vi "Motors Modular Bk.vi"(0 "Enable Motors":refnum<vi>, 1 "Cluster":T1, 2 "Motors Visa Ref":refnum<visa-resource-name>="COM7") -> ()   [LabVIEW 2010]
panel:
  in  "Enable Motors":bool
  out "Theta Action":string
  out "Z Action":string
  out "Y Action":string
  out "X Action":string
  in  "Steps to deactivate hard limit after finding datums":dbl=1000.0
  out "Loop i":i32
types:
  T1 = cluster{"Stop X?":refnum<vi>, "Stop Y?":refnum<vi>, "Stop Z?":refnum<vi>, "Stop Theta?":refnum<vi>, "Backlash?":refnum<vi>, "Backlash X":refnum<vi>, "Backlash Y":refnum<vi>, "Backlash Z":refnum<vi>, "Backlash Theta":refnum<vi>, "Manual IO?":refnum<vi>, "Manual Communication is Active\n(Close Before Ending Program)":refnum<vi>, "Reset Motors?":refnum<vi>, "Set Jogger?":refnum<vi>, "Normal":refnum<vi>, "Fast":refnum<vi>, "Jogger Axis":refnum<vi>, "Redefine Origin as Current Location?":refnum<vi>, "Save Current Motor Parameters?":refnum<vi>, "Find Datums Nearest Hard Limits?":refnum<vi>, "Saved Limits":refnum<vi>, "Use Datums Nearest Hard Limits to Reset Origin?":refnum<vi>, "X Go?":refnum<vi>, "Y Go?":refnum<vi>, "Z Go?":refnum<vi>, "Theta Go?":refnum<vi>, "Jog-Mode":refnum<vi>, "x+?":refnum<vi>, "x-?":refnum<vi>, "y+?":refnum<vi>, "y-?":refnum<vi>, "z+?":refnum<vi>, "z-?":refnum<vi>, "theta+?":refnum<vi>, "theta-?":refnum<vi>, "X Set Slew Speed?":refnum<vi>, "(mm/s)":refnum<vi>, "Y Set Slew Speed?":refnum<vi>, "(mm/s)":refnum<vi>, "Z Set Slew Speed?":refnum<vi>, "(mm/s)":refnum<vi>, "Theta Set Slew Speed?":refnum<vi>, "(degrees/s)":refnum<vi>, "Go To Saved Position?":refnum<vi>, "Defined Positions":refnum<vi>, "Need to Update Motor Parameters":refnum<vi>, "X Jogger Normal Speed":refnum<vi>, "X Jogger Fast Speed":refnum<vi>, "Y Jogger Normal Speed":refnum<vi>, "Y Jogger Fast Speed":refnum<vi>, "Z Jogger Normal Speed":refnum<vi>, "Z Jogger Fast Speed":refnum<vi>, "Theta Jogger Normal Speed":refnum<vi>, "Theta Jogger Fast Speed":refnum<vi>, "X Moving":refnum<vi>, "Y Moving":refnum<vi>, "Z Moving":refnum<vi>, "Theta Moving":refnum<vi>, "X Slew Speed (mm or degree/s)":refnum<vi>, "Y Slew Speed (mm or degree/s)":refnum<vi>, "Z Slew Speed (mm or degree/s)":refnum<vi>, "Theta Slew Speed (mm or degree/s)":refnum<vi>, "X-Axis (mm)":refnum<vi>, "Y-Axis (mm)":refnum<vi>, "Z-Axis (mm)":refnum<vi>, "Theta (deg)":refnum<vi>, "X Multiplier":refnum<vi>, "Y Multiplier":refnum<vi>, "Z Multiplier":refnum<vi>, "Theta Multiplier":refnum<vi>, "Motors Online":refnum<vi>, "Motors Status":refnum<vi>, "Status X":refnum<vi>, "Status Y":refnum<vi>, "Status Z":refnum<vi>, "Status Theta":refnum<vi>, "Motors error":refnum<vi>, "QUIT":refnum<vi>, "EMERGENCY":refnum<vi>, "X Go To":refnum<vi>, "Y Go To":refnum<vi>, "Z Go To":refnum<vi>, "Theta Go To":refnum<vi>, "Delta X (mm)":refnum<vi>, "Delta Y (mm)":refnum<vi>, "Delta Z (mm)":refnum<vi>, "Delta Theta (deg)":refnum<vi>, "X Speed (mm/s)":refnum<vi>, "Y Speed (mm/s)":refnum<vi>, "Z Speed (mm/s)":refnum<vi>, "Theta Speed (deg/s)":refnum<vi>, "x+":refnum<vi>, "x-":refnum<vi>, "y+":refnum<vi>, "y-":refnum<vi>, "z+":refnum<vi>, "z-":refnum<vi>, "theta+":refnum<vi>, "theta-":refnum<vi>, "Saved Positions":refnum<vi>}
  T2 = cluster{"Stop X?":refnum<vi>, "Stop Y?":refnum<vi>, "Stop Z?":refnum<vi>, "Stop Theta?":refnum<vi>}
  T3 = cluster{"Backlash?":refnum<vi>, "Backlash X":refnum<vi>, "Backlash Y":refnum<vi>, "Backlash Z":refnum<vi>, "Backlash Theta":refnum<vi>}
  T4 = cluster{"EMERGENCY":refnum<vi>, "Manual IO?":refnum<vi>, "Manual Communication is Active\n(Close Before Ending Program)":refnum<vi>, "Reset Motors?":refnum<vi>}
  T5 = cluster{"Redefine Origin as Current Location?":refnum<vi>, "Save Current Motor Parameters?":refnum<vi>}
  T6 = cluster{"X Set Slew Speed?":refnum<vi>, "(mm/s)":refnum<vi>, "Y Set Slew Speed?":refnum<vi>, "(mm/s)":refnum<vi>, "Z Set Slew Speed?":refnum<vi>, "(mm/s)":refnum<vi>, "Theta Set Slew Speed?":refnum<vi>, "(degrees/s)":refnum<vi>, "Need to Update Motor Parameters":refnum<vi>, "X Multiplier":refnum<vi>, "Y Multiplier":refnum<vi>, "Z Multiplier":refnum<vi>, "Theta Multiplier":refnum<vi>}
  T7 = cluster{"Set Jogger?":refnum<vi>, "Normal":refnum<vi>, "Fast":refnum<vi>, "Jogger Axis":refnum<vi>, "X Multiplier":refnum<vi>, "Y Multiplier":refnum<vi>, "Z Multiplier":refnum<vi>, "Theta Multiplier":refnum<vi>, "Need to Update Motor Parameters":refnum<vi>}
  T8 = cluster{"Need to Update Motor Parameters":refnum<vi>, "X Jogger Normal Speed":refnum<vi>, "X Jogger Fast Speed":refnum<vi>, "X Slew Speed (mm or degree/s)":refnum<vi>, "X-Axis (mm)":refnum<vi>, "Status X":refnum<vi>, "X Moving":refnum<vi>}
  T9 = cluster{"Y Slew Speed (mm or degree/s)":refnum<vi>, "Y Jogger Normal Speed":refnum<vi>, "Y Jogger Fast Speed":refnum<vi>, "Y-Axis (mm)":refnum<vi>, "Status Y":refnum<vi>, "Y Moving":refnum<vi>}
  T10 = cluster{"Z Slew Speed (mm or degree/s)":refnum<vi>, "Z Jogger Normal Speed":refnum<vi>, "Z Jogger Fast Speed":refnum<vi>, "Z-Axis (mm)":refnum<vi>, "Status Z":refnum<vi>, "Z Moving":refnum<vi>}
  T11 = cluster{"Theta Slew Speed (mm or degree/s)":refnum<vi>, "Theta Jogger Normal Speed":refnum<vi>, "Theta Jogger Fast Speed":refnum<vi>, "Theta (deg)":refnum<vi>, "Status Theta":refnum<vi>, "Theta Moving":refnum<vi>}
  T12 = cluster{"Find Datums Nearest Hard Limits?":refnum<vi>, "X Multiplier":refnum<vi>, "Y Multiplier":refnum<vi>, "Z Multiplier":refnum<vi>, "Theta Multiplier":refnum<vi>, "X-Axis (mm)":refnum<vi>, "Y-Axis (mm)":refnum<vi>, "Z-Axis (mm)":refnum<vi>, "Theta (deg)":refnum<vi>, "Status X":refnum<vi>, "Status Y":refnum<vi>, "Status Z":refnum<vi>, "Status Theta":refnum<vi>, "X Moving":refnum<vi>, "Y Moving":refnum<vi>, "Z Moving":refnum<vi>, "Theta Moving":refnum<vi>, "Saved Limits":refnum<vi>}
  T13 = cluster{"Status X":refnum<vi>, "X-Axis (mm)":refnum<vi>, "X Multiplier":refnum<vi>, "X Moving":refnum<vi>, "Status Y":refnum<vi>, "Y-Axis (mm)":refnum<vi>, "Y Multiplier":refnum<vi>, "Y Moving":refnum<vi>, "Status Z":refnum<vi>, "Z-Axis (mm)":refnum<vi>, "Z Multiplier":refnum<vi>, "Z Moving":refnum<vi>, "Status Theta":refnum<vi>, "Theta (deg)":refnum<vi>, "Theta Multiplier":refnum<vi>, "Theta Moving":refnum<vi>}
  T14 = cluster{"Use Datums Nearest Hard Limits to Reset Origin?":refnum<vi>, "X Multiplier":refnum<vi>, "Y Multiplier":refnum<vi>, "Z Multiplier":refnum<vi>, "Theta Multiplier":refnum<vi>, "X-Axis (mm)":refnum<vi>, "Y-Axis (mm)":refnum<vi>, "Z-Axis (mm)":refnum<vi>, "Theta (deg)":refnum<vi>, "Status X":refnum<vi>, "Status Y":refnum<vi>, "Status Z":refnum<vi>, "Status Theta":refnum<vi>}
  T15 = cluster{"X Go?":refnum<vi>, "X Multiplier":refnum<vi>, "X Go To":refnum<vi>, "Y Go?":refnum<vi>, "Y Multiplier":refnum<vi>, "Y Go To":refnum<vi>, "Z Go?":refnum<vi>, "Z Multiplier":refnum<vi>, "Z Go To":refnum<vi>, "Theta Go?":refnum<vi>, "Theta Multiplier":refnum<vi>, "Theta Go To":refnum<vi>}
  T16 = cluster{"Jog-Mode":refnum<vi>, "x+?":refnum<vi>, "x-?":refnum<vi>, "X Moving":refnum<vi>, "X Multiplier":refnum<vi>, "Delta X (mm)":refnum<vi>, "X Speed (mm/s)":refnum<vi>, "x+":refnum<vi>, "x-":refnum<vi>, "X-Axis (mm)":refnum<vi>, "Status X":refnum<vi>}
  T17 = cluster{"Jog-Mode":refnum<vi>, "y+?":refnum<vi>, "y-?":refnum<vi>, "Y Moving":refnum<vi>, "Delta Y (mm)":refnum<vi>, "Y Multiplier":refnum<vi>, "y+":refnum<vi>, "y-":refnum<vi>, "Y-Axis (mm)":refnum<vi>, "Status Y":refnum<vi>, "Y Speed (mm/s)":refnum<vi>}
  T18 = cluster{"Go To Saved Position?":refnum<vi>, "Defined Positions":refnum<vi>, "X Multiplier":refnum<vi>, "Y Multiplier":refnum<vi>, "Z Multiplier":refnum<vi>, "Theta Multiplier":refnum<vi>, "Saved Positions":refnum<vi>}
  T19 = cluster{"Jog-Mode":refnum<vi>, "z+?":refnum<vi>, "z-?":refnum<vi>, "Z Speed (mm/s)":refnum<vi>, "Delta Z (mm)":refnum<vi>, "Z Multiplier":refnum<vi>, "Z-Axis (mm)":refnum<vi>, "Status Z":refnum<vi>, "z+":refnum<vi>, "z-":refnum<vi>, "Z Moving":refnum<vi>}
  T20 = cluster{"Jog-Mode":refnum<vi>, "theta+?":refnum<vi>, "theta-?":refnum<vi>, "Theta Speed (deg/s)":refnum<vi>, "Delta Theta (deg)":refnum<vi>, "Theta Multiplier":refnum<vi>, "Theta (deg)":refnum<vi>, "Status Theta":refnum<vi>, "theta+":refnum<vi>, "theta-":refnum<vi>, "Theta Moving":refnum<vi>}
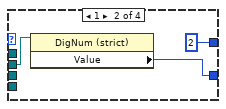
[diagram p3: hidden frame]
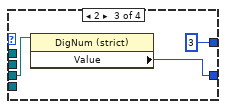
[diagram p4: hidden frame]
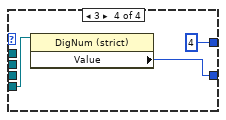
[diagram p5: hidden frame]
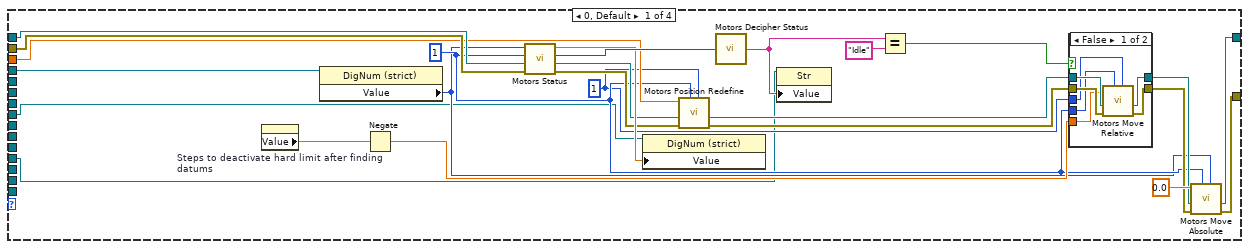
[diagram p15: hidden frame]
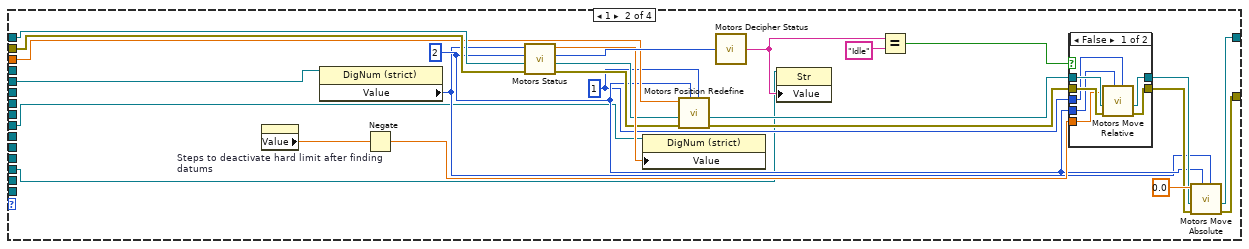
[diagram p17: hidden frame]
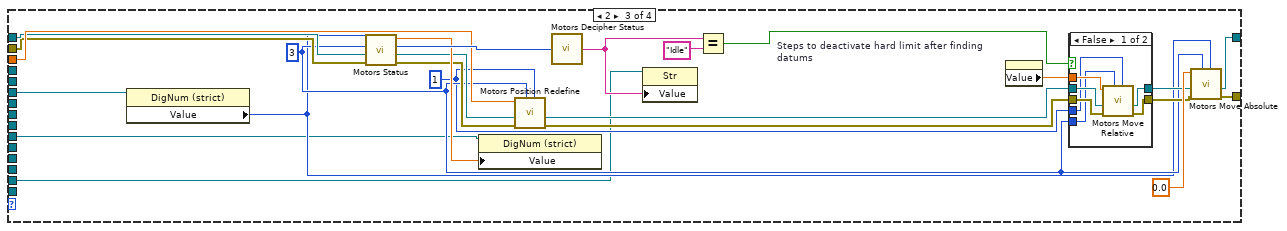
[diagram p19: hidden frame]
diagram:
  n1 = call "Motors Open.vi"("VISA in"="Motors Visa Ref") -> ("error out"=w130:errorcluster, "VISA out"=w127:refnum<visa-resource-name>)  [unwired: 1 in]
  n2 = call <vilib>:"Simple Error Handler.vi"("error in (no error)"=w130) -> ("error?"=w129:bool, "error out"=w131:errorcluster)  [unwired: 4 in, 3 out]
  n3 = Not(x=w129) -> (.not. x?=w128:bool)
  n4 = Unbundle("Cluster") -> ("Stop X?"=w122:refnum<vi>, "Stop Y?"=w121:refnum<vi>, "Stop Z?"=w120:refnum<vi>, "Stop Theta?"=w119:refnum<vi>, "Backlash?"=w118:refnum<vi>, "Backlash X"=w117:refnum<vi>, "Backlash Y"=w116:refnum<vi>, "Backlash Z"=w115:refnum<vi>, "Backlash Theta"=w114:refnum<vi>, "Manual IO?"=w112:refnum<vi>, "Manual Communication is Active\n(Close Before Ending Program)"=w111:refnum<vi>, "Reset Motors?"=w110:refnum<vi>, "Set Jogger?"=w106:refnum<vi>, "Normal"=w105:refnum<vi>, "Fast"=w104:refnum<vi>, "Jogger Axis"=w103:refnum<vi>, "Redefine Origin as Current Location?"=w101:refnum<vi>, "Save Current Motor Parameters?"=w100:refnum<vi>, "Find Datums Nearest Hard Limits?"=w98:refnum<vi>, "Saved Limits"=w93:refnum<vi>, "Use Datums Nearest Hard Limits to Reset Origin?"=w94:refnum<vi>, "X Go?"=w91:refnum<vi>, "Y Go?"=w89:refnum<vi>, "Z Go?"=w87:refnum<vi>, "Theta Go?"=w85:refnum<vi>, "Jog-Mode"=w63:refnum<vi>, "x+?"=w82:refnum<vi>, "x-?"=w81:refnum<vi>, "y+?"=w75:refnum<vi>, "y-?"=w74:refnum<vi>, "z+?"=w69:refnum<vi>, "z-?"=w68:refnum<vi>, "theta+?"=w62:refnum<vi>, "theta-?"=w61:refnum<vi>, "X Set Slew Speed?"=w53:refnum<vi>, "(mm/s)"=w52:refnum<vi>, "Y Set Slew Speed?"=w51:refnum<vi>, "(mm/s)"=w50:refnum<vi>, "Z Set Slew Speed?"=w49:refnum<vi>, "(mm/s)"=w48:refnum<vi>, "Theta Set Slew Speed?"=w47:refnum<vi>, "(degrees/s)"=w46:refnum<vi>, "Go To Saved Position?"=w43:refnum<vi>, "Defined Positions"=w42:refnum<vi>, "Need to Update Motor Parameters"=w34:refnum<vi>, "X Jogger Normal Speed"=w33:refnum<vi>, "X Jogger Fast Speed"=w32:refnum<vi>, "Y Jogger Normal Speed"=w25:refnum<vi>, "Y Jogger Fast Speed"=w24:refnum<vi>, "Z Jogger Normal Speed"=w18:refnum<vi>, "Z Jogger Fast Speed"=w17:refnum<vi>, "Theta Jogger Normal Speed"=w11:refnum<vi>, "Theta Jogger Fast Speed"=w10:refnum<vi>, "X Moving"=w29:refnum<vi>, "Y Moving"=w21:refnum<vi>, "Z Moving"=w14:refnum<vi>, "Theta Moving"=w7:refnum<vi>, "X Slew Speed (mm or degree/s)"=w28:refnum<vi>, "Y Slew Speed (mm or degree/s)"=w26:refnum<vi>, "Z Slew Speed (mm or degree/s)"=w19:refnum<vi>, "Theta Slew Speed (mm or degree/s)"=w12:refnum<vi>, "X-Axis (mm)"=w31:refnum<vi>, "Y-Axis (mm)"=w23:refnum<vi>, "Z-Axis (mm)"=w16:refnum<vi>, "Theta (deg)"=w9:refnum<vi>, "X Multiplier"=w41:refnum<vi>, "Y Multiplier"=w39:refnum<vi>, "Z Multiplier"=w38:refnum<vi>, "Theta Multiplier"=w40:refnum<vi>, "Motors Online"=w95:refnum<vi>, "Motors Status"=w97:refnum<vi>, "Status X"=w30:refnum<vi>, "Status Y"=w22:refnum<vi>, "Status Z"=w15:refnum<vi>, "Status Theta"=w8:refnum<vi>, "Motors error"=w2:refnum<vi>, "QUIT"=w126:refnum<vi>, "EMERGENCY"=w109:refnum<vi>, "X Go To"=w90:refnum<vi>, "Y Go To"=w88:refnum<vi>, "Z Go To"=w86:refnum<vi>, "Theta Go To"=w84:refnum<vi>, "Delta X (mm)"=w80:refnum<vi>, "Delta Y (mm)"=w73:refnum<vi>, "Delta Z (mm)"=w66:refnum<vi>, "Delta Theta (deg)"=w59:refnum<vi>, "X Speed (mm/s)"=w79:refnum<vi>, "Y Speed (mm/s)"=w70:refnum<vi>, "Z Speed (mm/s)"=w67:refnum<vi>, "Theta Speed (deg/s)"=w60:refnum<vi>, "x+"=w78:refnum<vi>, "x-"=w77:refnum<vi>, "y+"=w72:refnum<vi>, "y-"=w71:refnum<vi>, "z+"=w65:refnum<vi>, "z-"=w64:refnum<vi>, "theta+"=w58:refnum<vi>, "theta-"=w57:refnum<vi>, "Saved Positions"=w35:refnum<vi>)
  n5 = Bundle("Stop X?"=w122, "Stop Y?"=w121, "Stop Z?"=w120, "Stop Theta?"=w119) -> (w108:T2)  [unwired: 1 in]
  n6 = Bundle("Backlash?"=w118, "Backlash X"=w117, "Backlash Y"=w116, "Backlash Z"=w115, "Backlash Theta"=w114) -> (w113:T3)  [unwired: 1 in]
  n7 = property on="Property Node" class="Clust (strict)"(reference=w2, "Value"=w131) -> ()  [unwired: 1 in, 2 out]
  n8 = Bundle("EMERGENCY"=w109, "Manual IO?"=w112, "Manual Communication is Active\n(Close Before Ending Program)"=w111, "Reset Motors?"=w110) -> (w107:T4)  [unwired: 1 in]
  n9 = Bundle("Redefine Origin as Current Location?"=w101, "Save Current Motor Parameters?"=w100) -> (w99:T5)  [unwired: 1 in]
  n10 = Bundle("X Set Slew Speed?"=w53, "(mm/s)"=w52, "Y Set Slew Speed?"=w51, "(mm/s)"=w50, "Z Set Slew Speed?"=w49, "(mm/s)"=w48, "Theta Set Slew Speed?"=w47, "(degrees/s)"=w46, "Need to Update Motor Parameters"=w34, "X Multiplier"=w41, "Y Multiplier"=w39, "Z Multiplier"=w38, "Theta Multiplier"=w40) -> (w45:T6)  [unwired: 1 in]
  n11 = Bundle("Set Jogger?"=w106, "Normal"=w105, "Fast"=w104, "Jogger Axis"=w103, "X Multiplier"=w41, "Y Multiplier"=w39, "Z Multiplier"=w38, "Theta Multiplier"=w40, "Need to Update Motor Parameters"=w34) -> (w102:T7)  [unwired: 1 in]
  n12 = Bundle("Need to Update Motor Parameters"=w34, "X Jogger Normal Speed"=w33, "X Jogger Fast Speed"=w32, "X Slew Speed (mm or degree/s)"=w28, "X-Axis (mm)"=w31, "Status X"=w30, "X Moving"=w29) -> (w27:T8)  [unwired: 1 in]
  n13 = Bundle("Y Slew Speed (mm or degree/s)"=w26, "Y Jogger Normal Speed"=w25, "Y Jogger Fast Speed"=w24, "Y-Axis (mm)"=w23, "Status Y"=w22, "Y Moving"=w21) -> (w20:T9)  [unwired: 1 in]
  n14 = Bundle("Z Slew Speed (mm or degree/s)"=w19, "Z Jogger Normal Speed"=w18, "Z Jogger Fast Speed"=w17, "Z-Axis (mm)"=w16, "Status Z"=w15, "Z Moving"=w14) -> (w13:T10)  [unwired: 1 in]
  n15 = Bundle("Theta Slew Speed (mm or degree/s)"=w12, "Theta Jogger Normal Speed"=w11, "Theta Jogger Fast Speed"=w10, "Theta (deg)"=w9, "Status Theta"=w8, "Theta Moving"=w7) -> (w6:T11)  [unwired: 1 in]
  n16 = Bundle("Find Datums Nearest Hard Limits?"=w98, "X Multiplier"=w41, "Y Multiplier"=w39, "Z Multiplier"=w38, "Theta Multiplier"=w40, "X-Axis (mm)"=w31, "Y-Axis (mm)"=w23, "Z-Axis (mm)"=w16, "Theta (deg)"=w9, "Status X"=w30, "Status Y"=w22, "Status Z"=w15, "Status Theta"=w8, "X Moving"=w29, "Y Moving"=w21, "Z Moving"=w14, "Theta Moving"=w7, "Saved Limits"=w93) -> (w96:T12)  [unwired: 1 in]
  n17 = Bundle("Status X"=w30, "X-Axis (mm)"=w31, "X Multiplier"=w41, "X Moving"=w29, "Status Y"=w22, "Y-Axis (mm)"=w23, "Y Multiplier"=w39, "Y Moving"=w21, "Status Z"=w15, "Z-Axis (mm)"=w16, "Z Multiplier"=w38, "Z Moving"=w14, "Status Theta"=w8, "Theta (deg)"=w9, "Theta Multiplier"=w40, "Theta Moving"=w7) -> (w44:T13)  [unwired: 1 in]
  n18 = Bundle("Use Datums Nearest Hard Limits to Reset Origin?"=w94, "X Multiplier"=w41, "Y Multiplier"=w39, "Z Multiplier"=w38, "Theta Multiplier"=w40, "X-Axis (mm)"=w31, "Y-Axis (mm)"=w23, "Z-Axis (mm)"=w16, "Theta (deg)"=w9, "Status X"=w30, "Status Y"=w22, "Status Z"=w15, "Status Theta"=w8) -> (w92:T14)  [unwired: 1 in]
  n19 = Bundle("X Go?"=w91, "X Multiplier"=w41, "X Go To"=w90, "Y Go?"=w89, "Y Multiplier"=w39, "Y Go To"=w88, "Z Go?"=w87, "Z Multiplier"=w38, "Z Go To"=w86, "Theta Go?"=w85, "Theta Multiplier"=w40, "Theta Go To"=w84) -> (w83:T15)  [unwired: 1 in]
  n20 = Bundle("Jog-Mode"=w63, "x+?"=w82, "x-?"=w81, "X Moving"=w29, "X Multiplier"=w41, "Delta X (mm)"=w80, "X Speed (mm/s)"=w79, "x+"=w78, "x-"=w77, "X-Axis (mm)"=w31, "Status X"=w30) -> (w76:T16)  [unwired: 1 in]
  n21 = Bundle("Jog-Mode"=w63, "y+?"=w75, "y-?"=w74, "Y Moving"=w21, "Delta Y (mm)"=w73, "Y Multiplier"=w39, "y+"=w72, "y-"=w71, "Y-Axis (mm)"=w23, "Status Y"=w22, "Y Speed (mm/s)"=w70) -> (w56:T17)  [unwired: 1 in]
  n22 = Bundle("Go To Saved Position?"=w43, "Defined Positions"=w42, "X Multiplier"=w41, "Y Multiplier"=w39, "Z Multiplier"=w38, "Theta Multiplier"=w40, "Saved Positions"=w35) -> (w37:T18)  [unwired: 1 in]
  n23 = Bundle("Jog-Mode"=w63, "z+?"=w69, "z-?"=w68, "Z Speed (mm/s)"=w67, "Delta Z (mm)"=w66, "Z Multiplier"=w38, "Z-Axis (mm)"=w16, "Status Z"=w15, "z+"=w65, "z-"=w64, "Z Moving"=w14) -> (w55:T19)  [unwired: 1 in]
  n24 = Bundle("Jog-Mode"=w63, "theta+?"=w62, "theta-?"=w61, "Theta Speed (deg/s)"=w60, "Delta Theta (deg)"=w59, "Theta Multiplier"=w40, "Theta (deg)"=w9, "Status Theta"=w8, "theta+"=w58, "theta-"=w57, "Theta Moving"=w7) -> (w54:T20)  [unwired: 1 in]
  n25 = property on="Property Node" class="Bool (strict)"(reference=w95, "Value"=w128) -> ()  [unwired: 1 in, 2 out]
  n26 = property on="Property Node" class="Str"(reference=w97, "Value"="Opening Communications") -> (reference out=w125:refnum<vi>)  [unwired: 1 in, 1 out]
  n27 = property on="Property Node" class="Bool (strict)"(reference=w34, "Value"=TRUE) -> ()  [unwired: 1 in, 2 out]
  n28 = case shown="True" w128 {
    tunnel: w125 -> [_ w158]
    tunnel: w127 -> [w133 w157]
    tunnel: w2 -> [_ w156]
    tunnel: w126 -> [_ w155]
    tunnel: w113 -> [_ w135]
    tunnel: w108 -> [_ w153]
    tunnel: w107 -> [_ w152]
    tunnel: w102 -> [_ w151]
    tunnel: w99 -> [_ w150]
    tunnel: w96 -> [_ w149]
    tunnel: w92 -> [_ w148]
    tunnel: w83 -> [_ w147]
    tunnel: w76 -> [_ w146]
    tunnel: w56 -> [_ w145]
    tunnel: w55 -> [_ w144]
    tunnel: w54 -> [_ w143]
    tunnel: w45 -> [_ w142]
    tunnel: w44 -> [_ w141]
    tunnel: w37 -> [_ w140]
    tunnel: w27 -> [_ w139]
    tunnel: w20 -> [_ w138]
    tunnel: w13 -> [_ w137]
    tunnel: w6 -> [_ w136]
    tunnel: [w133 w134] -> w5
    frame False {
    }
    frame True {
      n29 = property on="Property Node" class="Str"(reference=w158, "Value"="Running") -> (reference out=w154:refnum<vi>)  [unwired: 1 in, 1 out]
      n30 = while {
        shift-right: [w167] -> w134
        shift-left: w157 -> [w395]
        tunnel: w156 -> [w165]
        tunnel: w155 -> [w439]
        tunnel: w154 -> [w436]
        tunnel: w135 -> [w384]
        tunnel: w153 -> [w396]
        tunnel: w152 -> [w373]
        tunnel: w151 -> [w355]
        tunnel: w150 -> [w354]
        tunnel: w149 -> [w349]
        tunnel: w148 -> [w330]
        tunnel: w147 -> [w316]
        tunnel: w146 -> [w303]
        tunnel: w145 -> [w289]
        tunnel: w144 -> [w274]
        tunnel: w143 -> [w261]
        tunnel: w142 -> [w247]
        tunnel: w141 -> [w225]
        tunnel: w140 -> [w208]
        tunnel: w139 -> [w197]
        tunnel: w138 -> [w188]
        tunnel: w137 -> [w181]
        tunnel: w136 -> [w174]
        i -> [w440]
        stop <- w163 stop-if-true
        # "This loop contains all of the code that has to communicate directly with the manipulator motor controllers.  They are arranged linearly to ensure multiple serial I/O's are never attempted simultaneously.  Note that this loop executes very slowly (each serial I/O takes about 1/20 sec).\n\nWarning: Pushing LabView's \"Clean Up Diagram\" button will likely cause LabView to crash (because this VI is way too big)."
        n31 = Unbundle(w396) -> ("Stop X?"=w411:refnum<vi>, "Stop Y?"=w412:refnum<vi>, "Stop Z?"=w413:refnum<vi>, "Stop Theta?"=w414:refnum<vi>)
        n32 = property on="Property Node" class="Bool (strict)"(reference=w439) -> ("Value"=w164:bool)  [unwired: 1 in, 2 out]
        n33 = property on="Property Node" class="Bool (strict)"(reference=w411) -> (reference out=w410:refnum<vi>, "Value"=w403:bool)  [unwired: 1 in, 1 out]
        n34 = property on="Property Node" class="Clust (strict)"(reference=w165) -> (reference out=w166:refnum<vi>, "Value"=w394:errorcluster)  [unwired: 1 in, 1 out]
        n35 = property on="Property Node" class="Bool (strict)"(reference="Enable Motors") -> ("Value"=w161:bool)  [unwired: 1 in, 2 out]
        n36 = Not(x=w161) -> (.not. x?=w160:bool)
        n37 = Or(x=w164, y=w160) -> (x .or. y?=w163:bool)
        n38 = case shown="True" w403 {
          tunnel: w394 -> [w597 w605]
          tunnel: w395 -> [w598 w604]
          tunnel: [w598 w602] -> w402
          tunnel: [w597 w601] -> w401
          tunnel: w410 -> [_ w599]
          frame False {
          }
          frame True {
            n39 = property on="Property Node" class="Bool (strict)"(reference=w599, "Value"=FALSE) -> ()  [unwired: 1 in, 2 out]
            n40 = call "Motors Stop.vi"("error in"=w605, "Axis"=1, "VISA in"=w604) -> ("error out"=w601:errorcluster, "VISA out"=w602:refnum<visa-resource-name>)
          }
        }
        n41 = property on="Property Node" class="Bool (strict)"(reference=w412) -> (reference out=w409:refnum<vi>, "Value"=w404:bool)  [unwired: 1 in, 1 out]
        n42 = case shown="True" w404 {
          tunnel: w401 -> [w588 w596]
          tunnel: w402 -> [w589 w595]
          tunnel: [w589 w593] -> w400
          tunnel: [w588 w592] -> w399
          tunnel: w409 -> [_ w590]
          frame False {
          }
          frame True {
            n43 = property on="Property Node" class="Bool (strict)"(reference=w590, "Value"=FALSE) -> ()  [unwired: 1 in, 2 out]
            n44 = call "Motors Stop.vi"("error in"=w596, "Axis"=2, "VISA in"=w595) -> ("error out"=w592:errorcluster, "VISA out"=w593:refnum<visa-resource-name>)
          }
        }
        n45 = property on="Property Node" class="Bool (strict)"(reference=w413) -> (reference out=w408:refnum<vi>, "Value"=w405:bool)  [unwired: 1 in, 1 out]
        n46 = case shown="True" w405 {
          tunnel: w399 -> [w579 w587]
          tunnel: w400 -> [w580 w586]
          tunnel: [w580 w584] -> w398
          tunnel: [w579 w583] -> w397
          tunnel: w408 -> [_ w581]
          frame False {
          }
          frame True {
            n47 = property on="Property Node" class="Bool (strict)"(reference=w581, "Value"=FALSE) -> ()  [unwired: 1 in, 2 out]
            n48 = call "Motors Stop.vi"("error in"=w587, "Axis"=3, "VISA in"=w586) -> ("error out"=w583:errorcluster, "VISA out"=w584:refnum<visa-resource-name>)
          }
        }
        n49 = property on="Property Node" class="Bool (strict)"(reference=w414) -> (reference out=w407:refnum<vi>, "Value"=w406:bool)  [unwired: 1 in, 1 out]
        n50 = case shown="True" w406 {
          tunnel: w397 -> [w570 w578]
          tunnel: w398 -> [w571 w577]
          tunnel: [w571 w575] -> w385
          tunnel: [w570 w574] -> w386
          tunnel: w407 -> [_ w572]
          frame False {
          }
          frame True {
            n51 = property on="Property Node" class="Bool (strict)"(reference=w572, "Value"=FALSE) -> ()  [unwired: 1 in, 2 out]
            n52 = call "Motors Stop.vi"("error in"=w578, "Axis"=4, "VISA in"=w577) -> ("error out"=w574:errorcluster, "VISA out"=w575:refnum<visa-resource-name>)
          }
        }
        n53 = Unbundle(w384) -> ("Backlash?"=w391:refnum<vi>, "Backlash X"=w387:refnum<vi>, "Backlash Y"=w388:refnum<vi>, "Backlash Z"=w389:refnum<vi>, "Backlash Theta"=w390:refnum<vi>)
        n54 = property on="Property Node" class="Bool (strict)"(reference=w391) -> (reference out=w393:refnum<vi>, "Value"=w392:bool)  [unwired: 1 in, 1 out]
        n55 = case shown="True" w392 {
          tunnel: [w555 w569] -> w372
          tunnel: w387 -> [_ w568]
          tunnel: w388 -> [_ w566]
          tunnel: w389 -> [_ w564]
          tunnel: w390 -> [_ w562]
          tunnel: w393 -> [_ w559]
          tunnel: w385 -> [w555 w558]
          tunnel: w386 -> [w554 w557]
          tunnel: [w554 w556] -> w371
          frame False {
          }
          frame True {
            n56 = property on="Property Node" class="Bool (strict)"(reference=w559, "Value"=FALSE) -> ()  [unwired: 1 in, 2 out]
            n57 = property on="Property Node" class="DigNum (strict)"(reference=w568) -> ("Value"=w567:u32)  [unwired: 1 in, 2 out]
            n58 = property on="Property Node" class="DigNum (strict)"(reference=w566) -> ("Value"=w565:u32)  [unwired: 1 in, 2 out]
            n59 = property on="Property Node" class="DigNum (strict)"(reference=w564) -> ("Value"=w563:u32)  [unwired: 1 in, 2 out]
            n60 = property on="Property Node" class="DigNum (strict)"(reference=w562) -> ("Value"=w561:u32)  [unwired: 1 in, 2 out]
            n61 = call "Motors Backlash.vi"("X"=w567, "Y"=w565, "VISA in"=w558, "error in"=w557, "Z"=w563, "Theta"=w561) -> ("VISA out"=w569:refnum<visa-resource-name>, "error out"=w556:errorcluster)  [unwired: 2 in]
          }
        }
        n62 = Unbundle(w373) -> ("EMERGENCY"=w376:refnum<vi>, "Manual IO?"=w379:refnum<vi>, "Manual Communication is Active\n(Close Before Ending Program)"=w377:refnum<vi>, "Reset Motors?"=w381:refnum<vi>)
        n63 = property on="Property Node" class="Bool (strict)"(reference=w379) -> (reference out=w380:refnum<vi>, "Value"=w378:bool)  [unwired: 1 in, 1 out]
        n64 = case shown="True" w378 {
          tunnel: [w527 w540] -> w375
          tunnel: [w528 w530] -> w374
          tunnel: w376 -> [_ w537]
          tunnel: w377 -> [_ w536]
          tunnel: w380 -> [_ w532]
          tunnel: w372 -> [w528 w531]
          tunnel: w371 -> [w527 w529]
          frame False {
          }
          frame True {
            n65 = property on="Property Node" class="Bool (strict)"(reference=w532, "Value"=FALSE) -> ()  [unwired: 1 in, 2 out]
            n66 = flat-sequence {
              tunnel: w536 -> [w542]
              tunnel: [w541] -> w534
              tunnel: [w549] -> w539
              tunnel: [w548] -> w538
              tunnel: w537 -> [w547]
              tunnel: [w546] -> w535
              tunnel: w534 -> [w546]
              tunnel: w531 -> [w545]
              tunnel: w529 -> [w544]
              tunnel: [w552] -> w530
              tunnel: [w553] -> w540
              tunnel: w539 -> [w553]
              tunnel: w538 -> [w552]
              tunnel: w535 -> [w550]
              frame #0 {
                n67 = property on="Property Node" class="Bool (strict)"(reference=w542, "Value"=TRUE ("Manual Communication is Active\n(Close Before Ending Program) 2")) -> (reference out=w541:refnum<vi>)  [unwired: 1 in, 1 out]
              }
              frame #1 {
                n68 = call "Motors Manual IO.vi"("error in"=w544, "Emergency Stop Reference"=w547, "VISA in"=w545) -> ("error out"=w549:errorcluster, "VISA out"=w548:refnum<visa-resource-name>)
              }
              frame #2 {
                n69 = property on="Property Node" class="Bool (strict)"(reference=w550, "Value"=FALSE ("Manual Communication is Active\n(Close Before Ending Program)")) -> ()  [unwired: 1 in, 2 out]
              }
            }
          }
        }
        n70 = Unbundle(w355) -> ("Set Jogger?"=w358:refnum<vi>, "Normal"=w360:refnum<vi>, "Fast"=w361:refnum<vi>, "Jogger Axis"=w364:refnum<vi>, "X Multiplier"=w366:refnum<vi>, "Y Multiplier"=w367:refnum<vi>, "Z Multiplier"=w368:refnum<vi>, "Theta Multiplier"=w369:refnum<vi>, "Need to Update Motor Parameters"=w370:refnum<vi>)
        n71 = property on="Property Node" class="Ring (strict)"(reference=w364) -> ("Value"=w365:u16)  [unwired: 1 in, 2 out]
        n72 = property on="Property Node" class="Bool (strict)"(reference=w381) -> (reference out=w383:refnum<vi>, "Value"=w382:bool)  [unwired: 1 in, 1 out]
        n73 = case shown="0, Default" w365 {
          tunnel: [u32 1 u32 2 u32 3 u32 4] -> _
          tunnel: [w493 w496 w499 w502] -> w363
          tunnel: w366 -> [w492 _ _ _]
          tunnel: w367 -> [_ w495 _ _]
          tunnel: w369 -> [_ _ _ w501]
          tunnel: w368 -> [_ _ w498 _]
          frame 0, Default {
            n74 = property on="Property Node" class="DigNum (strict)"(reference=w492) -> ("Value"=w493:u32)  [unwired: 1 in, 2 out]
          }
          frame 1 {
            n75 = property on="Property Node" class="DigNum (strict)"(reference=w495) -> ("Value"=w496:u32)  [unwired: 1 in, 2 out]
          }
          frame 2 {
            n76 = property on="Property Node" class="DigNum (strict)"(reference=w498) -> ("Value"=w499:u32)  [unwired: 1 in, 2 out]
          }
          frame 3 {
            n77 = property on="Property Node" class="DigNum (strict)"(reference=w501) -> ("Value"=w502:u32)  [unwired: 1 in, 2 out]
          }
        }
        n78 = case shown="True" w382 {
          tunnel: [w519 w526] -> w356
          tunnel: [w520 w525] -> w357
          tunnel: w374 -> [w520 w524]
          tunnel: w375 -> [w519 w523]
          tunnel: w383 -> [_ w521]
          frame False {
          }
          frame True {
            n79 = property on="Property Node" class="Bool (strict)"(reference=w521, "Value"=FALSE) -> ()  [unwired: 1 in, 2 out]
            n80 = call "Motors Reset.vi"("error in"=w523, "VISA in"=w524) -> ("error out"=w526:errorcluster, "VISA out"=w525:refnum<visa-resource-name>)
          }
        }
        n81 = property on="Property Node" class="Bool (strict)"(reference=w358) -> (reference out=w362:refnum<vi>, "Value"=w359:bool)  [unwired: 1 in, 1 out]
        n82 = case shown="True" w359 {
          tunnel: [w505 w518] -> w351
          tunnel: [w504 w516] -> w352
          tunnel: w363 -> [_ w517]
          tunnel: w362 -> [_ w514]
          tunnel: w360 -> [_ w510]
          tunnel: w361 -> [_ w509]
          tunnel: w356 -> [w505 w508]
          tunnel: w357 -> [w504 w507]
          tunnel: w370 -> [_ w506]
          frame False {
          }
          frame True {
            n83 = property on="Property Node" class="Bool (strict)"(reference=w514, "Value"=FALSE ("Need to Update Motor Parameters")) -> ()  [unwired: 1 in, 2 out]
            n84 = property on="Property Node" class="Bool (strict)"(reference=w506, "Value"=TRUE) -> ()  [unwired: 1 in, 2 out]
            n85 = property on="Property Node" class="DigNum (strict)"(reference=w510) -> ("Value"=w513:dbl)  [unwired: 1 in, 2 out]
            n86 = property on="Property Node" class="DigNum (strict)"(reference=w509) -> ("Value"=w512:dbl)  [unwired: 1 in, 2 out]
            n87 = call "Motors Jogger Speed.vi"("Axis Multiplier"=w517, "error in"=w508, "VISA in"=w507, "Fast Speed (mm or degree/sec)"=w512, "Normal Speed (mm or degree/sec)"=w513) -> ("error out"=w518:errorcluster, "VISA out"=w516:refnum<visa-resource-name>)  [unwired: 5 in]
          }
        }
        n88 = Unbundle(w354) -> ("Redefine Origin as Current Location?"=w353:refnum<vi>, "Save Current Motor Parameters?"=w350:refnum<vi>)
        n89 = property on="Property Node" class="Bool (strict)"(reference=w350) -> (reference out=w428:refnum<vi>, "Value"=w427:bool)  [unwired: 1 in, 1 out]
        n90 = property on="Property Node" class="Bool (strict)"(reference=w353) -> (reference out=w426:refnum<vi>, "Value"=w438:bool)  [unwired: 1 in, 1 out]
        n91 = case shown="True" w438 {
          tunnel: w352 -> [w1796 w1803]
          tunnel: w351 -> [w1797 w1799]
          tunnel: [w1797 w1801] -> w429
          tunnel: [w1796 w1802] -> w491
          tunnel: w426 -> [_ w1798]
          frame False {
          }
          frame True {
            n92 = property on="Property Node" class="Bool (strict)"(reference=w1798, "Value"=FALSE) -> ()  [unwired: 1 in, 2 out]
            n93 = call "Motors Redefine Origin.vi"("error in"=w1799, "VISA in"=w1803) -> ("error out"=w1801:errorcluster, "VISA out"=w1802:refnum<visa-resource-name>)
          }
        }
        n94 = case shown="True" w427 {
          tunnel: w429 -> [w1789 w1795]
          tunnel: [w1789 w1794] -> w446
          tunnel: w491 -> [w1788 w1793]
          tunnel: [w1788 w1792] -> w445
          tunnel: w428 -> [_ w1791]
          frame False {
          }
          frame True {
            n95 = property on="Property Node" class="Bool (strict)"(reference=w1791, "Value"=FALSE) -> ()  [unwired: 1 in, 2 out]
            n96 = call "Motors Save.vi"("error in"=w1795, "VISA in"=w1793) -> ("error out"=w1794:errorcluster, "VISA out"=w1792:refnum<visa-resource-name>)
          }
        }
        n97 = Unbundle(w349) -> ("Find Datums Nearest Hard Limits?"=w348:refnum<vi>, "X Multiplier"=w347:refnum<vi>, "Y Multiplier"=w346:refnum<vi>, "Z Multiplier"=w345:refnum<vi>, "Theta Multiplier"=w344:refnum<vi>, "X-Axis (mm)"=w343:refnum<vi>, "Y-Axis (mm)"=w342:refnum<vi>, "Z-Axis (mm)"=w341:refnum<vi>, "Theta (deg)"=w340:refnum<vi>, "Status X"=w339:refnum<vi>, "Status Y"=w338:refnum<vi>, "Status Z"=w337:refnum<vi>, "Status Theta"=w336:refnum<vi>, "X Moving"=w335:refnum<vi>, "Y Moving"=w334:refnum<vi>, "Z Moving"=w333:refnum<vi>, "Theta Moving"=w332:refnum<vi>, "Saved Limits"=w331:refnum<vi>)
        n98 = property on="Property Node" class="Bool (strict)"(reference=w348) -> (reference out=w431:refnum<vi>, "Value"=w437:bool)  [unwired: 1 in, 1 out]
        n99 = case shown="True" w437 {
          tunnel: w446 -> [w823 w854]
          tunnel: [w823 w852] -> w443
          tunnel: [w822 w853] -> w441
          tunnel: w445 -> [w822 w855]
          tunnel: w436 -> [w821 w847]
          tunnel: [w820 w844] -> w434
          tunnel: [w821 w843] -> w433
          tunnel: w431 -> [_ w842]
          tunnel: w347 -> [_ w840]
          tunnel: w346 -> [_ w839]
          tunnel: w345 -> [_ w838]
          tunnel: w344 -> [_ w837]
          tunnel: w343 -> [_ w836]
          tunnel: w342 -> [_ w835]
          tunnel: w341 -> [_ w834]
          tunnel: w340 -> [_ w833]
          tunnel: w339 -> [_ w832]
          tunnel: w338 -> [_ w831]
          tunnel: w337 -> [_ w830]
          tunnel: w336 -> [_ w829]
          tunnel: w335 -> [_ w828]
          tunnel: w334 -> [_ w827]
          tunnel: w333 -> [_ w826]
          tunnel: w332 -> [_ w825]
          tunnel: w331 -> [w820 w824]
          frame False {
          }
          frame True {
            n100 = property on="Property Node" class="Bool (strict)"(reference=w842, "Value"=FALSE) -> ()  [unwired: 1 in, 2 out]
            n101 = flat-sequence {
              tunnel: w854 -> [w860]
              tunnel: w855 -> [w861]
              tunnel: [w861] -> w851
              tunnel: [w860] -> w850
              tunnel: w847 -> [w857]
              tunnel: [w856] -> w845
              tunnel: w851 -> [w897]
              tunnel: w850 -> [w896]
              tunnel: [w892] -> w849
              tunnel: [w891] -> w848
              tunnel: [w881] -> w846
              tunnel: w845 -> [w881]
              tunnel: [w879] -> w844
              tunnel: w840 -> [w878]
              tunnel: w839 -> [w877]
              tunnel: w838 -> [w876]
              tunnel: w837 -> [w875]
              tunnel: w836 -> [w874]
              tunnel: w835 -> [w873]
              tunnel: w834 -> [w872]
              tunnel: w833 -> [w871]
              tunnel: w832 -> [w870]
              tunnel: w831 -> [w869]
              tunnel: w830 -> [w868]
              tunnel: w829 -> [w867]
              tunnel: w828 -> [w866]
              tunnel: w827 -> [w865]
              tunnel: w826 -> [w864]
              tunnel: w825 -> [w863]
              tunnel: w824 -> [w862]
              tunnel: [w1007] -> w852
              tunnel: [w1008] -> w853
              tunnel: w849 -> [w1008]
              tunnel: w848 -> [w1007]
              tunnel: w846 -> [w1005]
              tunnel: [w1004] -> w843
              frame #0 {
                n102 = call <vilib>:"Set Busy.vi"("disable click? (T)"=FALSE) -> ()  [unwired: 9 in, 2 out]
                n103 = property on="Property Node" class="Str"(reference=w857, "Value"="Finding Datums Nearest Hard Limits\nThis May Take a Few Minutes" ("Status")) -> (reference out=w856:refnum<vi>)  [unwired: 1 in, 1 out]
              }
              frame #1 {
                n104 = call "Motors Find Datums.vi"("error in"=w896, "VISA in"=w897) -> ("error out"=w893:errorcluster, "VISA out"=w894:refnum<visa-resource-name>)
                n105 = for {
                  N: 4 -> [_]
                  shift-right: [w917] -> w891
                  shift-left: w893 -> [w918]
                  shift-right: [w916] -> w892
                  shift-left: w894 -> [w919]
                  tunnel: [w915] -> w883 mode=indexing
                  tunnel: w878 -> [w913]
                  tunnel: w877 -> [w912]
                  tunnel: w876 -> [w911]
                  tunnel: w875 -> [w910]
                  tunnel: w874 -> [w909]
                  tunnel: w873 -> [w908]
                  tunnel: w872 -> [w907]
                  tunnel: w871 -> [w906]
                  tunnel: w870 -> [w905]
                  tunnel: w869 -> [w904]
                  tunnel: w868 -> [w903]
                  tunnel: w867 -> [w902]
                  tunnel: w866 -> [w901]
                  tunnel: w865 -> [w900]
                  tunnel: w864 -> [w899]
                  tunnel: w863 -> [w898]
                  i -> [w914]
                  n106 = case shown="0, Default" w914 {
                    tunnel: w918 -> [w932 w953 w974 w995]
                    tunnel: w919 -> [w933 w954 w975 w996]
                    tunnel: [w926 w947 w967 w988] -> w917
                    tunnel: [w927 w948 w968 w989] -> w916
                    tunnel: [w924 w945 w971 w992] -> w915
                    tunnel: w913 -> [w923 _ _ _]
                    tunnel: w912 -> [_ w944 _ _]
                    tunnel: w911 -> [_ _ w965 _]
                    tunnel: w910 -> [_ _ _ w986]
                    tunnel: w909 -> [w922 _ _ _]
                    tunnel: w908 -> [_ w943 _ _]
                    tunnel: w907 -> [_ _ w964 _]
                    tunnel: w906 -> [_ _ _ w985]
                    tunnel: w905 -> [w921 _ _ _]
                    tunnel: w904 -> [_ w942 _ _]
                    tunnel: w903 -> [_ _ w963 _]
                    tunnel: w902 -> [_ _ _ w984]
                    tunnel: w901 -> [w920 _ _ _]
                    tunnel: w900 -> [_ w941 _ _]
                    tunnel: w899 -> [_ _ w962 _]
                    tunnel: w898 -> [_ _ _ w983]
                    frame 0, Default {
                      w925 = 1 ("Axis")
                      n107 = property on="Property Node" class="DigNum (strict)"(reference=w923) -> ("Value"=w931:u32)  [unwired: 1 in, 2 out]
                      n108 = call "Motors Status.vi"("error in"=w932, "VISA in"=w933, "Axis"=w925, "Axis Multiplier"=w931) -> ("error out"=w928:errorcluster, "VISA out"=w929:refnum<visa-resource-name>, "OS"=w938:i32, "Actual Position (mm or deg)"=w930:dbl)  [unwired: 3 in]
                      n109 = property on="Property Node" class="DigNum (strict)"(reference=w922, "Value"=w930) -> ()  [unwired: 1 in, 2 out]
                      n110 = call "Motors Datum Position.vi"("error in"=w928, "VISA in"=w929, "Axis"=w925) -> ("error out"=w926:errorcluster, "VISA out"=w927:refnum<visa-resource-name>, "Datum Position (steps)"=w924:string)  [unwired: 5 in]
                      n111 = call "Motors Decipher Status.vi"("OS"=w938) -> ("Status"=w937:string)
                      n112 = property on="Property Node" class="Str"(reference=w921, "Value"=w937) -> ()  [unwired: 1 in, 2 out]
                      n113 = Equal?(x=w937, y="Idle") -> (x = y?=w935:bool)
                      n114 = case shown="False" w935 {
                        tunnel: [TRUE FALSE] -> w934
                        frame False {
                        }
                        frame True {
                        }
                      }
                      n115 = property on="Property Node" class="Bool (strict)"(reference=w920, "Value"=w934) -> ()  [unwired: 1 in, 2 out]
                    }
                    frame 1 {
                      w946 = 2 ("Axis")
                      n116 = property on="Property Node" class="DigNum (strict)"(reference=w944) -> ("Value"=w952:u32)  [unwired: 1 in, 2 out]
                      n117 = call "Motors Status.vi"("error in"=w953, "VISA in"=w954, "Axis"=w946, "Axis Multiplier"=w952) -> ("error out"=w949:errorcluster, "VISA out"=w950:refnum<visa-resource-name>, "OS"=w959:i32, "Actual Position (mm or deg)"=w951:dbl)  [unwired: 3 in]
                      n118 = property on="Property Node" class="DigNum (strict)"(reference=w943, "Value"=w951) -> ()  [unwired: 1 in, 2 out]
                      n119 = call "Motors Datum Position.vi"("error in"=w949, "VISA in"=w950, "Axis"=w946) -> ("error out"=w947:errorcluster, "VISA out"=w948:refnum<visa-resource-name>, "Datum Position (steps)"=w945:string)  [unwired: 5 in]
                      n120 = call "Motors Decipher Status.vi"("OS"=w959) -> ("Status"=w957:string)
                      n121 = property on="Property Node" class="Str"(reference=w942, "Value"=w957) -> ()  [unwired: 1 in, 2 out]
                      n122 = Equal?(x=w957, y="Idle") -> (x = y?=w956:bool)
                      n123 = case shown="False" w956 {
                        tunnel: [TRUE FALSE] -> w955
                        frame False {
                        }
                        frame True {
                        }
                      }
                      n124 = property on="Property Node" class="Bool (strict)"(reference=w941, "Value"=w955) -> ()  [unwired: 1 in, 2 out]
                    }
                    frame 2 {
                      w966 = 3 ("Axis")
                      n125 = property on="Property Node" class="DigNum (strict)"(reference=w965) -> ("Value"=w973:u32)  [unwired: 1 in, 2 out]
                      n126 = call "Motors Status.vi"("error in"=w974, "VISA in"=w975, "Axis"=w966, "Axis Multiplier"=w973) -> ("error out"=w969:errorcluster, "VISA out"=w970:refnum<visa-resource-name>, "OS"=w980:i32, "Actual Position (mm or deg)"=w972:dbl)  [unwired: 3 in]
                      n127 = property on="Property Node" class="DigNum (strict)"(reference=w964, "Value"=w972) -> ()  [unwired: 1 in, 2 out]
                      n128 = call "Motors Datum Position.vi"("error in"=w969, "VISA in"=w970, "Axis"=w966) -> ("error out"=w967:errorcluster, "VISA out"=w968:refnum<visa-resource-name>, "Datum Position (steps)"=w971:string)  [unwired: 5 in]
                      n129 = call "Motors Decipher Status.vi"("OS"=w980) -> ("Status"=w978:string)
                      n130 = property on="Property Node" class="Str"(reference=w963, "Value"=w978) -> ()  [unwired: 1 in, 2 out]
                      n131 = Equal?(x=w978, y="Idle") -> (x = y?=w977:bool)
                      n132 = case shown="False" w977 {
                        tunnel: [TRUE FALSE] -> w976
                        frame False {
                        }
                        frame True {
                        }
                      }
                      n133 = property on="Property Node" class="Bool (strict)"(reference=w962, "Value"=w976) -> ()  [unwired: 1 in, 2 out]
                    }
                    frame 3 {
                      w987 = 4 ("Axis")
                      n134 = property on="Property Node" class="DigNum (strict)"(reference=w986) -> ("Value"=w994:u32)  [unwired: 1 in, 2 out]
                      n135 = call "Motors Status.vi"("error in"=w995, "VISA in"=w996, "Axis"=w987, "Axis Multiplier"=w994) -> ("error out"=w990:errorcluster, "VISA out"=w991:refnum<visa-resource-name>, "OS"=w1001:i32, "Actual Position (mm or deg)"=w993:dbl)  [unwired: 3 in]
                      n136 = property on="Property Node" class="DigNum (strict)"(reference=w985, "Value"=w993) -> ()  [unwired: 1 in, 2 out]
                      n137 = call "Motors Datum Position.vi"("error in"=w990, "VISA in"=w991, "Axis"=w987) -> ("error out"=w988:errorcluster, "VISA out"=w989:refnum<visa-resource-name>, "Datum Position (steps)"=w992:string)  [unwired: 5 in]
                      n138 = call "Motors Decipher Status.vi"("OS"=w1001) -> ("Status"=w999:string)
                      n139 = property on="Property Node" class="Str"(reference=w984, "Value"=w999) -> ()  [unwired: 1 in, 2 out]
                      n140 = Equal?(x=w999, y="Idle") -> (x = y?=w998:bool)
                      n141 = case shown="True" w998 {
                        tunnel: [TRUE FALSE] -> w997
                        frame False {
                        }
                        frame True {
                        }
                      }
                      n142 = property on="Property Node" class="Bool (strict)"(reference=w983, "Value"=w997) -> ()  [unwired: 1 in, 2 out]
                    }
                  }
                }
                n143 = Build Array (concatenate)("Limits", w883) -> (w882:string[])
                n144 = Initialize Array("", 0 ("dimension size"), 0 ("dimension size")) -> (w889:string[][])
                n145 = Build Array (concatenate)(w882, w889) -> (w887:string[][])
                n146 = property on="Property Node" class="Path"(reference=w862) -> (reference out=w879:refnum<vi>, "Value"=w880:path)  [unwired: 1 in, 1 out]
                n147 = Transpose 2D Array(2D array=w887) -> (transposed array=w886:string[][])
                n148 = call "Motors Position Rewrite.vi"("file path"=w880, "Array of Positions"=w886) -> ()  [unwired: 9 in]
              }
              frame #2 {
                n149 = call <vilib>:"Unset Busy.vi"() -> ()  [unwired: 11 in, 1 out]
                n150 = property on="Property Node" class="Str"(reference=w1005, "Value"="Running" ("Status")) -> (reference out=w1004:refnum<vi>)  [unwired: 1 in, 1 out]
              }
            }
          }
        }
        n151 = Unbundle(w330) -> ("Use Datums Nearest Hard Limits to Reset Origin?"=w329:refnum<vi>, "X Multiplier"=w328:refnum<vi>, "Y Multiplier"=w327:refnum<vi>, "Z Multiplier"=w326:refnum<vi>, "Theta Multiplier"=w325:refnum<vi>, "X-Axis (mm)"=w324:refnum<vi>, "Y-Axis (mm)"=w323:refnum<vi>, "Z-Axis (mm)"=w322:refnum<vi>, "Theta (deg)"=w321:refnum<vi>, "Status X"=w320:refnum<vi>, "Status Y"=w319:refnum<vi>, "Status Z"=w318:refnum<vi>, "Status Theta"=w317:refnum<vi>)
        n152 = property on="Property Node" class="Bool (strict)"(reference=w329) -> (reference out=w430:refnum<vi>, "Value"=w435:bool)  [unwired: 1 in, 1 out]
        n153 = case shown="True" w435 {
          tunnel: [w608 w629] -> w444
          tunnel: w443 -> [w608 w631]
          tunnel: [w607 w628] -> w442
          tunnel: w441 -> [w607 w632]
          tunnel: w434 -> [_ w627]
          tunnel: w433 -> [w606 w623]
          tunnel: [w606 w624] -> w198
          tunnel: w430 -> [_ w622]
          tunnel: w328 -> [_ w620]
          tunnel: w327 -> [_ w619]
          tunnel: w326 -> [_ w618]
          tunnel: w325 -> [_ w617]
          tunnel: w324 -> [_ w616]
          tunnel: w323 -> [_ w615]
          tunnel: w322 -> [_ w614]
          tunnel: w321 -> [_ w613]
          tunnel: w320 -> [_ w612]
          tunnel: w319 -> [_ w611]
          tunnel: w318 -> [_ w610]
          tunnel: w317 -> [_ w609]
          frame False {
          }
          frame True {
            n154 = property on="Property Node" class="Bool (strict)"(reference=w622, "Value"=FALSE) -> ()  [unwired: 1 in, 2 out]
            n155 = flat-sequence {
              tunnel: w631 -> [w636]
              tunnel: [w636] -> w630
              tunnel: w623 -> [w634]
              tunnel: [w633] -> w625
              tunnel: w632 -> [w660]
              tunnel: w630 -> [w661]
              tunnel: [w656] -> w629
              tunnel: [w655] -> w628
              tunnel: w627 -> [w651]
              tunnel: [w649] -> w626
              tunnel: w625 -> [w649]
              tunnel: w620 -> [w648]
              tunnel: w619 -> [w647]
              tunnel: w618 -> [w646]
              tunnel: w617 -> [w645]
              tunnel: w616 -> [w644]
              tunnel: w615 -> [w643]
              tunnel: w614 -> [w642]
              tunnel: w613 -> [w641]
              tunnel: w612 -> [w640]
              tunnel: w611 -> [w639]
              tunnel: w610 -> [w638]
              tunnel: w609 -> [w637]
              tunnel: w626 -> [w818]
              tunnel: [w817] -> w624
              frame #0 {
                n156 = call <vilib>:"Set Busy.vi"() -> ()  [unwired: 10 in, 2 out]
                n157 = property on="Property Node" class="Str"(reference=w634, "Value"="Finding Datums Nearest Hard Limits\nThis May Take a Few Minutes" ("Status")) -> (reference out=w633:refnum<vi>)  [unwired: 1 in, 1 out]
              }
              frame #1 {
                n158 = property on="Property Node" class="Path"(reference=w651) -> ("Value"=w650:path)  [unwired: 1 in, 2 out]
                n159 = call "Motors Find Datums.vi"("error in"=w661, "VISA in"=w660) -> ("error out"=w658:errorcluster, "VISA out"=w659:refnum<visa-resource-name>)
                n160 = call "Motors Position Load.vi"("error in"=w658, "file path"=w650) -> ("error out"=w657:errorcluster, "Positions"=w654:string[][])
                n161 = Delete From Array(array=w654, index (row)=0) -> (array with subset deleted=w652:string[][])  [unwired: 2 in, 1 out]
                n162 = for {
                  shift-right: [w680] -> w656
                  shift-left: w657 -> [w681]
                  shift-right: [w679] -> w655
                  shift-left: w659 -> [w682]
                  tunnel: w652 -> [w678] mode=indexing
                  tunnel: w648 -> [w673]
                  tunnel: w647 -> [w672]
                  tunnel: w646 -> [w671]
                  tunnel: w645 -> [w670]
                  tunnel: w644 -> [w669]
                  tunnel: w643 -> [w668]
                  tunnel: w642 -> [w667]
                  tunnel: w641 -> [w666]
                  tunnel: w640 -> [w665]
                  tunnel: w639 -> [w664]
                  tunnel: w638 -> [w663]
                  tunnel: w637 -> [w662]
                  i -> [w675]
                  n163 = Index Array(array=w678, index=0) -> (element=w677:string)
                  n164 = Fract/Exp String To Number(string=w677) -> (number=w676:dbl)  [unwired: 3 in, 1 out]
                  n165 = case shown="3" w675 {
                    tunnel: w681 -> [w702 w736 w766 w802]
                    tunnel: w682 -> [w703 w737 w767 w803]
                    tunnel: [w696 w729 w758 w795] -> w680
                    tunnel: [w697 w730 w759 w796] -> w679
                    tunnel: w676 -> [w698 w732 w769 w798]
                    tunnel: w673 -> [w685 _ _ _]
                    tunnel: w672 -> [_ w719 _ _]
                    tunnel: w671 -> [_ _ w753 _]
                    tunnel: w670 -> [_ _ _ w786]
                    tunnel: w669 -> [w684 _ _ _]
                    tunnel: w668 -> [_ w718 _ _]
                    tunnel: w667 -> [_ _ w752 _]
                    tunnel: w666 -> [_ _ _ w785]
                    tunnel: w665 -> [w683 _ _ _]
                    tunnel: w664 -> [_ w717 _ _]
                    tunnel: w663 -> [_ _ w751 _]
                    tunnel: w662 -> [_ _ _ w784]
                    frame 0, Default {
                      w686 = u32 1 ("Axis Multiplier")
                      w688 = 1 ("Axis")
                      n166 = property on="Steps to deactivate hard limit after finding datums" class="DigNum (strict)"() -> ("Value"=w694:dbl)  [unwired: 2 in, 2 out]
                      n167 = property on="Property Node" class="DigNum (strict)"(reference=w685) -> ("Value"=w687:u32)  [unwired: 1 in, 2 out]
                      n168 = Negate(x=w694) -> (-x=w689:dbl)
                      n169 = call "Motors Status.vi"("error in"=w702, "VISA in"=w703, "Axis"=w688, "Axis Multiplier"=w687) -> ("error out"=w699:errorcluster, "VISA out"=w700:refnum<visa-resource-name>, "OS"=w707:i32, "Actual Position (mm or deg)"=w701:dbl)  [unwired: 3 in]
                      n170 = property on="Property Node" class="DigNum (strict)"(reference=w684, "Value"=w701) -> ()  [unwired: 1 in, 2 out]
                      n171 = call "Motors Position Redefine.vi"("Axis Multiplier"=w686, "Axis"=w688, "error in"=w699, "VISA in"=w700, "Position (mm or deg)"=w698) -> ("error out"=w693:errorcluster, "VISA out"=w690:refnum<visa-resource-name>)  [unwired: 5 in]
                      n172 = call "Motors Decipher Status.vi"("OS"=w707) -> ("Status"=w706:string)
                      n173 = property on="Property Node" class="Str"(reference=w683, "Value"=w706) -> ()  [unwired: 1 in, 2 out]
                      n174 = Equal?(x=w706, y="Idle") -> (x = y?=w704:bool)
                      n175 = case shown="False" w704 {
                        tunnel: w693 -> [w714 w716]
                        tunnel: [w713 w716] -> w692
                        tunnel: w690 -> [w712 w715]
                        tunnel: [w711 w715] -> w691
                        tunnel: w689 -> [w710 _]
                        tunnel: w688 -> [w709 _]
                        tunnel: w686 -> [w708 _]
                        frame False {
                          n176 = call "Motors Move Relative.vi"("Axis Multiplier"=w708, "Axis"=w709, "error in"=w714, "VISA in"=w712, "Distance (mm)"=w710) -> ("error out"=w713:errorcluster, "VISA out"=w711:refnum<visa-resource-name>)  [unwired: 5 in]
                        }
                        frame True {
                        }
                      }
                      n177 = call "Motors Move Absolute.vi"("Axis Multiplier"=w687, "Axis"=w688, "error in"=w692, "VISA in"=w691, "Position (mm or degree)"=0.0) -> ("error out"=w696:errorcluster, "VISA out"=w697:refnum<visa-resource-name>)  [unwired: 5 in]
                    }
                    frame 1 {
                      w720 = u32 1 ("Axis Multiplier")
                      w722 = 2 ("Axis")
                      n178 = property on="Steps to deactivate hard limit after finding datums" class="DigNum (strict)"() -> ("Value"=w728:dbl)  [unwired: 2 in, 2 out]
                      n179 = property on="Property Node" class="DigNum (strict)"(reference=w719) -> ("Value"=w721:u32)  [unwired: 1 in, 2 out]
                      n180 = Negate(x=w728) -> (-x=w723:dbl)
                      n181 = call "Motors Status.vi"("error in"=w736, "VISA in"=w737, "Axis"=w722, "Axis Multiplier"=w721) -> ("error out"=w733:errorcluster, "VISA out"=w734:refnum<visa-resource-name>, "OS"=w741:i32, "Actual Position (mm or deg)"=w735:dbl)  [unwired: 3 in]
                      n182 = property on="Property Node" class="DigNum (strict)"(reference=w718, "Value"=w735) -> ()  [unwired: 1 in, 2 out]
                      n183 = call "Motors Position Redefine.vi"("Axis Multiplier"=w720, "Axis"=w722, "error in"=w733, "VISA in"=w734, "Position (mm or deg)"=w732) -> ("error out"=w726:errorcluster, "VISA out"=w727:refnum<visa-resource-name>)  [unwired: 5 in]
                      n184 = call "Motors Decipher Status.vi"("OS"=w741) -> ("Status"=w739:string)
                      n185 = property on="Property Node" class="Str"(reference=w717, "Value"=w739) -> ()  [unwired: 1 in, 2 out]
                      n186 = Equal?(x=w739, y="Idle") -> (x = y?=w738:bool)
                      n187 = case shown="False" w738 {
                        tunnel: w727 -> [w748 w749]
                        tunnel: w726 -> [w747 w750]
                        tunnel: [w746 w749] -> w725
                        tunnel: [w745 w750] -> w724
                        tunnel: w723 -> [w744 _]
                        tunnel: w722 -> [w743 _]
                        tunnel: w720 -> [w742 _]
                        frame False {
                          n188 = call "Motors Move Relative.vi"("Axis Multiplier"=w742, "Axis"=w743, "error in"=w747, "VISA in"=w748, "Distance (mm)"=w744) -> ("error out"=w745:errorcluster, "VISA out"=w746:refnum<visa-resource-name>)  [unwired: 5 in]
                        }
                        frame True {
                        }
                      }
                      n189 = call "Motors Move Absolute.vi"("Axis Multiplier"=w721, "Axis"=w722, "error in"=w724, "VISA in"=w725, "Position (mm or degree)"=0.0) -> ("error out"=w729:errorcluster, "VISA out"=w730:refnum<visa-resource-name>)  [unwired: 5 in]
                    }
                    frame 2 {
                      w754 = u32 1 ("Axis Multiplier")
                      w756 = 3 ("Axis")
                      n190 = property on="Property Node" class="DigNum (strict)"(reference=w753) -> ("Value"=w755:u32)  [unwired: 1 in, 2 out]
                      n191 = call "Motors Status.vi"("error in"=w766, "VISA in"=w767, "Axis"=w756, "Axis Multiplier"=w755) -> ("error out"=w764:errorcluster, "VISA out"=w765:refnum<visa-resource-name>, "OS"=w774:i32, "Actual Position (mm or deg)"=w770:dbl)  [unwired: 3 in]
                      n192 = property on="Property Node" class="DigNum (strict)"(reference=w752, "Value"=w770) -> ()  [unwired: 1 in, 2 out]
                      n193 = call "Motors Position Redefine.vi"("Axis Multiplier"=w754, "Axis"=w756, "error in"=w764, "VISA in"=w765, "Position (mm or deg)"=w769) -> ("error out"=w762:errorcluster, "VISA out"=w763:refnum<visa-resource-name>)  [unwired: 5 in]
                      n194 = call "Motors Decipher Status.vi"("OS"=w774) -> ("Status"=w772:string)
                      n195 = property on="Property Node" class="Str"(reference=w751, "Value"=w772) -> ()  [unwired: 1 in, 2 out]
                      n196 = Equal?(x=w772, y="Idle") -> (x = y?=w771:bool)
                      n197 = property on="Steps to deactivate hard limit after finding datums" class="DigNum (strict)"() -> ("Value"=w757:dbl)  [unwired: 2 in, 2 out]
                      n198 = case shown="False" w771 {
                        tunnel: w763 -> [w781 w782]
                        tunnel: w762 -> [w780 w783]
                        tunnel: [w779 w782] -> w761
                        tunnel: [w778 w783] -> w760
                        tunnel: w757 -> [w777 _]
                        tunnel: w756 -> [w776 _]
                        tunnel: w754 -> [w775 _]
                        frame False {
                          n199 = call "Motors Move Relative.vi"("Axis Multiplier"=w775, "Axis"=w776, "error in"=w780, "VISA in"=w781, "Distance (mm)"=w777) -> ("error out"=w778:errorcluster, "VISA out"=w779:refnum<visa-resource-name>)  [unwired: 5 in]
                        }
                        frame True {
                        }
                      }
                      n200 = call "Motors Move Absolute.vi"("Axis Multiplier"=w755, "Axis"=w756, "error in"=w760, "VISA in"=w761, "Position (mm or degree)"=0.0) -> ("error out"=w758:errorcluster, "VISA out"=w759:refnum<visa-resource-name>)  [unwired: 5 in]
                    }
                    frame 3 {
                      w787 = u32 1 ("Axis Multiplier")
                      w789 = 4 ("Axis")
                      n201 = property on="Property Node" class="DigNum (strict)"(reference=w786) -> ("Value"=w788:u32)  [unwired: 1 in, 2 out]
                      n202 = call "Motors Status.vi"("error in"=w802, "VISA in"=w803, "Axis"=w789, "Axis Multiplier"=w788) -> ("error out"=w799:errorcluster, "VISA out"=w800:refnum<visa-resource-name>, "OS"=w807:i32, "Actual Position (mm or deg)"=w801:dbl)  [unwired: 3 in]
                      n203 = property on="Property Node" class="DigNum (strict)"(reference=w785, "Value"=w801) -> ()  [unwired: 1 in, 2 out]
                      n204 = call "Motors Position Redefine.vi"("Axis Multiplier"=w787, "Axis"=w789, "error in"=w799, "VISA in"=w800, "Position (mm or deg)"=w798) -> ("error out"=w793:errorcluster, "VISA out"=w794:refnum<visa-resource-name>)  [unwired: 5 in]
                      n205 = call "Motors Decipher Status.vi"("OS"=w807) -> ("Status"=w805:string)
                      n206 = property on="Property Node" class="Str"(reference=w784, "Value"=w805) -> ()  [unwired: 1 in, 2 out]
                      n207 = Equal?(x=w805, y="Idle") -> (x = y?=w804:bool)
                      n208 = case shown="False" w804 {
                        tunnel: w794 -> [w814 w816]
                        tunnel: w793 -> [w813 w815]
                        tunnel: [w812 w816] -> w792
                        tunnel: [w811 w815] -> w791
                        tunnel: "Steps to deactivate hard limit after finding datums" -> [w810 _]
                        tunnel: w789 -> [w809 _]
                        tunnel: w787 -> [w808 _]
                        frame False {
                          n209 = call "Motors Move Relative.vi"("Axis Multiplier"=w808, "Axis"=w809, "error in"=w813, "VISA in"=w814, "Distance (mm)"=w810) -> ("error out"=w811:errorcluster, "VISA out"=w812:refnum<visa-resource-name>)  [unwired: 5 in]
                        }
                        frame True {
                        }
                      }
                      n210 = call "Motors Move Absolute.vi"("Axis Multiplier"=w788, "Axis"=w789, "error in"=w791, "VISA in"=w792, "Position (mm or degree)"=0.0) -> ("error out"=w795:errorcluster, "VISA out"=w796:refnum<visa-resource-name>)  [unwired: 5 in]
                    }
                  }
                }
              }
              frame #2 {
                n211 = call <vilib>:"Unset Busy.vi"() -> ()  [unwired: 11 in, 1 out]
                n212 = property on="Property Node" class="Str"(reference=w818, "Value"="Running" ("Status")) -> (reference out=w817:refnum<vi>)  [unwired: 1 in, 1 out]
              }
            }
          }
        }
        n213 = Unbundle(w316) -> ("X Go?"=w315:refnum<vi>, "X Multiplier"=w314:refnum<vi>, "X Go To"=w313:refnum<vi>, "Y Go?"=w312:refnum<vi>, "Y Multiplier"=w311:refnum<vi>, "Y Go To"=w310:refnum<vi>, "Z Go?"=w309:refnum<vi>, "Z Multiplier"=w308:refnum<vi>, "Z Go To"=w307:refnum<vi>, "Theta Go?"=w306:refnum<vi>, "Theta Multiplier"=w305:refnum<vi>, "Theta Go To"=w304:refnum<vi>)
        n214 = property on="Property Node" class="Bool (strict)"(reference=w315) -> (reference out=w419:refnum<vi>, "Value"=w432:bool)  [unwired: 1 in, 1 out]
        n215 = case shown="True" w432 {
          tunnel: w442 -> [w1776 w1784]
          tunnel: w444 -> [w1775 w1787]
          tunnel: [w1776 w1785] -> w490
          tunnel: [w1775 w1786] -> w489
          tunnel: w419 -> [_ w1782]
          tunnel: w314 -> [_ w1778]
          tunnel: w313 -> [_ w1777]
          frame False {
          }
          frame True {
            n216 = property on="Property Node" class="DigNum (strict)"(reference=w1778) -> ("Value"=w1780:u32)  [unwired: 1 in, 2 out]
            n217 = property on="Property Node" class="DigNum (strict)"(reference=w1777) -> ("Value"=w1779:dbl)  [unwired: 1 in, 2 out]
            n218 = property on="Property Node" class="Bool (strict)"(reference=w1782, "Value"=FALSE) -> ()  [unwired: 1 in, 2 out]
            n219 = call "Motors Move Absolute.vi"("Axis Multiplier"=w1780, "Axis"=u32 1, "error in"=w1787, "VISA in"=w1784, "Position (mm or degree)"=w1779) -> ("error out"=w1786:errorcluster, "VISA out"=w1785:refnum<visa-resource-name>)  [unwired: 5 in]
          }
        }
        n220 = property on="Property Node" class="Bool (strict)"(reference=w312) -> (reference out=w424:refnum<vi>, "Value"=w425:bool)  [unwired: 1 in, 1 out]
        n221 = case shown="True" w425 {
          tunnel: w490 -> [w1763 w1771]
          tunnel: w489 -> [w1762 w1774]
          tunnel: [w1763 w1772] -> w488
          tunnel: [w1762 w1773] -> w487
          tunnel: w424 -> [_ w1766]
          tunnel: w311 -> [_ w1765]
          tunnel: w310 -> [_ w1764]
          frame False {
          }
          frame True {
            n222 = property on="Property Node" class="DigNum (strict)"(reference=w1765) -> ("Value"=w1769:u32)  [unwired: 1 in, 2 out]
            n223 = property on="Property Node" class="DigNum (strict)"(reference=w1764) -> ("Value"=w1768:dbl)  [unwired: 1 in, 2 out]
            n224 = property on="Property Node" class="Bool (strict)"(reference=w1766, "Value"=FALSE) -> ()  [unwired: 1 in, 2 out]
            n225 = call "Motors Move Absolute.vi"("Axis Multiplier"=w1769, "Axis"=u32 2, "error in"=w1774, "VISA in"=w1771, "Position (mm or degree)"=w1768) -> ("error out"=w1773:errorcluster, "VISA out"=w1772:refnum<visa-resource-name>)  [unwired: 5 in]
          }
        }
        n226 = property on="Property Node" class="Bool (strict)"(reference=w309) -> (reference out=w422:refnum<vi>, "Value"=w423:bool)  [unwired: 1 in, 1 out]
        n227 = case shown="True" w423 {
          tunnel: w488 -> [w1750 w1756]
          tunnel: w487 -> [w1749 w1761]
          tunnel: [w1750 w1759] -> w486
          tunnel: [w1749 w1760] -> w485
          tunnel: w422 -> [_ w1753]
          tunnel: w308 -> [_ w1752]
          tunnel: w307 -> [_ w1751]
          frame False {
          }
          frame True {
            n228 = property on="Property Node" class="DigNum (strict)"(reference=w1752) -> ("Value"=w1757:u32)  [unwired: 1 in, 2 out]
            n229 = property on="Property Node" class="DigNum (strict)"(reference=w1751) -> ("Value"=w1755:dbl)  [unwired: 1 in, 2 out]
            n230 = property on="Property Node" class="Bool (strict)"(reference=w1753, "Value"=FALSE) -> ()  [unwired: 1 in, 2 out]
            n231 = call "Motors Move Absolute.vi"("Axis Multiplier"=w1757, "Axis"=u32 3, "error in"=w1761, "VISA in"=w1756, "Position (mm or degree)"=w1755) -> ("error out"=w1760:errorcluster, "VISA out"=w1759:refnum<visa-resource-name>)  [unwired: 5 in]
          }
        }
        n232 = property on="Property Node" class="Bool (strict)"(reference=w306) -> (reference out=w420:refnum<vi>, "Value"=w421:bool)  [unwired: 1 in, 1 out]
        n233 = case shown="True" w421 {
          tunnel: w486 -> [w1736 w1745]
          tunnel: w485 -> [w1737 w1748]
          tunnel: [w1737 w1747] -> w483
          tunnel: [w1736 w1746] -> w484
          tunnel: w420 -> [_ w1740]
          tunnel: w305 -> [_ w1739]
          tunnel: w304 -> [_ w1738]
          frame False {
          }
          frame True {
            n234 = property on="Property Node" class="DigNum (strict)"(reference=w1739) -> ("Value"=w1743:u32)  [unwired: 1 in, 2 out]
            n235 = property on="Property Node" class="DigNum (strict)"(reference=w1738) -> ("Value"=w1742:dbl)  [unwired: 1 in, 2 out]
            n236 = property on="Property Node" class="Bool (strict)"(reference=w1740, "Value"=FALSE) -> ()  [unwired: 1 in, 2 out]
            n237 = call "Motors Move Absolute.vi"("Axis Multiplier"=w1743, "Axis"=u32 4, "error in"=w1748, "VISA in"=w1745, "Position (mm or degree)"=w1742) -> ("error out"=w1747:errorcluster, "VISA out"=w1746:refnum<visa-resource-name>)  [unwired: 5 in]
          }
        }
        n238 = Unbundle(w303) -> ("Jog-Mode"=w300:refnum<vi>, "x+?"=w301:refnum<vi>, "x-?"=w302:refnum<vi>, "X Moving"=w291:refnum<vi>, "X Multiplier"=w296:refnum<vi>, "Delta X (mm)"=w290:refnum<vi>, "X Speed (mm/s)"=w297:refnum<vi>, "x+"=w293:refnum<vi>, "x-"=w292:refnum<vi>, "X-Axis (mm)"=w295:refnum<vi>, "Status X"=w294:refnum<vi>)
        n239 = property on="Property Node" class="Bool (strict)"(reference=w301) -> (reference out=w417:refnum<vi>, "Value"=w455:bool)  [unwired: 1 in, 1 out]
        n240 = property on="Property Node" class="Bool (strict)"(reference=w302) -> (reference out=w418:refnum<vi>, "Value"=w454:bool)  [unwired: 1 in, 1 out]
        n241 = property on="Property Node" class="Bool (strict)"(reference=w300) -> ("Value"=w298:bool)  [unwired: 1 in, 2 out]
        n242 = Or(x=w455, y=w454) -> (x .or. y?=w482:bool)
        n243 = case shown="True" w482 {
          tunnel: w484 -> [w1629 w1646]
          tunnel: w483 -> [w1628 w1645]
          tunnel: w298 -> [_ w1647]
          tunnel: [w1629 w1643] -> w481
          tunnel: [w1628 w1642] -> w480
          tunnel: w454 -> [_ w1644]
          tunnel: w418 -> [_ w1639]
          tunnel: w417 -> [_ w1638]
          tunnel: w297 -> [_ w1637]
          tunnel: w296 -> [_ w1636]
          tunnel: w295 -> [_ w1635]
          tunnel: w294 -> [_ w1634]
          tunnel: w293 -> [_ w1633]
          tunnel: w292 -> [_ w1632]
          tunnel: w291 -> [_ w1631]
          tunnel: w290 -> [_ w1630]
          frame False {
          }
          frame True {
            n244 = flat-sequence {
              tunnel: w1647 -> [w1661]
              tunnel: w1646 -> [w1660]
              tunnel: w1645 -> [w1659]
              tunnel: w1644 -> [w1658]
              tunnel: [w1657] -> w1641
              tunnel: [w1656] -> w1640
              tunnel: w1637 -> [w1655]
              tunnel: w1636 -> [w1654]
              tunnel: w1635 -> [w1653]
              tunnel: w1634 -> [w1652]
              tunnel: w1633 -> [w1651]
              tunnel: w1632 -> [w1650]
              tunnel: w1631 -> [w1649]
              tunnel: w1630 -> [w1648]
              tunnel: [w1734] -> w1642
              tunnel: [w1735] -> w1643
              tunnel: w1641 -> [w1735]
              tunnel: w1640 -> [w1734]
              tunnel: w1639 -> [w1731]
              tunnel: w1638 -> [w1730]
              frame #0 {
                n245 = case shown="False" w1661 {
                  tunnel: w1660 -> [w1671 w1701]
                  tunnel: w1659 -> [w1667 w1704]
                  tunnel: w1658 -> [w1670 w1709]
                  tunnel: [w1669 w1706] -> w1657
                  tunnel: [w1668 w1705] -> w1656
                  tunnel: w1655 -> [_ w1696]
                  tunnel: w1654 -> [w1662 w1695]
                  tunnel: w1653 -> [_ w1694]
                  tunnel: w1652 -> [_ w1693]
                  tunnel: w1651 -> [_ w1692]
                  tunnel: w1650 -> [_ w1691]
                  tunnel: w1649 -> [w1664 _]
                  tunnel: w1648 -> [w1663 _]
                  frame False {
                    n246 = property on="Property Node" class="Bool (strict)"(reference=w1664) -> (reference out=w1665:refnum<vi>, "Value"=w1666:bool)  [unwired: 1 in, 1 out]
                    n247 = case shown="False" w1666 {
                      tunnel: w1671 -> [w1679 w1690]
                      tunnel: w1667 -> [w1684 w1689]
                      tunnel: w1670 -> [w1683 _]
                      tunnel: [w1681 w1690] -> w1669
                      tunnel: [w1682 w1689] -> w1668
                      tunnel: w1665 -> [w1675 _]
                      tunnel: w1663 -> [w1673 _]
                      tunnel: w1662 -> [w1672 _]
                      frame False {
                        n248 = property on="Property Node" class="Bool (strict)"(reference=w1675, "Value"=TRUE ("X Moving")) -> ()  [unwired: 1 in, 2 out]
                        n249 = property on="Property Node" class="DigNum (strict)"(reference=w1672) -> ("Value"=w1677:u32)  [unwired: 1 in, 2 out]
                        n250 = property on="Property Node" class="DigNum (strict)"(reference=w1673) -> ("Value"=w1674:dbl)  [unwired: 1 in, 2 out]
                        n251 = case shown="True" w1683 {
                          tunnel: w1674 -> [w1685 w1687]
                          tunnel: [w1685 w1686] -> w1680
                          frame False {
                          }
                          frame True {
                            n252 = Multiply(x=w1687, y=-1.0) -> (x*y=w1686:dbl)
                          }
                        }
                        n253 = call "Motors Move Relative.vi"("Axis Multiplier"=w1677, "Axis"=1, "error in"=w1684, "VISA in"=w1679, "Distance (mm)"=w1680) -> ("error out"=w1682:errorcluster, "VISA out"=w1681:refnum<visa-resource-name>)  [unwired: 5 in]
                      }
                      frame True {
                      }
                    }
                  }
                  frame True {
                    w1698 = 1 ("Axis")
                    n254 = property on="Property Node" class="DigNum (strict)"(reference=w1695) -> ("Value"=w1699:u32)  [unwired: 1 in, 2 out]
                    n255 = property on="Property Node" class="DigNum (strict)"(reference=w1696) -> ("Value"=w1697:dbl)  [unwired: 1 in, 2 out]
                    n256 = case shown="True" w1709 {
                      tunnel: w1697 -> [w1726 w1728]
                      tunnel: [w1726 w1727] -> w1702
                      frame False {
                      }
                      frame True {
                        n257 = Multiply(x=w1728, y=-1.0) -> (x*y=w1727:dbl)
                      }
                    }
                    n258 = call "Motors Move Constant Velocity.vi"("Axis Multiplier"=w1699, "Axis"=w1698, "error in"=w1704, "VISA in"=w1701, "Speed (mm/s)"=w1702) -> ("error out"=w1703:errorcluster, "VISA out"=w1700:refnum<visa-resource-name>)  [unwired: 5 in]
                    n259 = while {
                      tunnel: w1700 -> [w1715]
                      tunnel: [w1717] -> w1708
                      tunnel: w1703 -> [w1718]
                      tunnel: [w1716] -> w1707
                      tunnel: w1699 -> [w1714]
                      tunnel: w1694 -> [w1713]
                      tunnel: w1693 -> [w1712]
                      tunnel: w1692 -> [w1711]
                      tunnel: w1691 -> [w1710]
                      stop <- w1723 continue-if-true
                      n260 = property on="Property Node" class="Bool (strict)"(reference=w1711) -> ("Value"=w1724:bool)  [unwired: 1 in, 2 out]
                      n261 = property on="Property Node" class="Bool (strict)"(reference=w1710) -> ("Value"=w1725:bool)  [unwired: 1 in, 2 out]
                      n262 = Or(x=w1724, y=w1725) -> (x .or. y?=w1723:bool)
                      n263 = call "Motors Status.vi"("error in"=w1718, "VISA in"=w1715, "Axis"=1, "Axis Multiplier"=w1714) -> ("error out"=w1716:errorcluster, "VISA out"=w1717:refnum<visa-resource-name>, "OS"=w1721:i32, "Actual Position (mm or deg)"=w1719:dbl)  [unwired: 3 in]
                      n264 = property on="Property Node" class="DigNum (strict)"(reference=w1713, "Value"=w1719) -> ()  [unwired: 1 in, 2 out]
                      n265 = call "Motors Decipher Status.vi"("OS"=w1721) -> ("Status"=w1720:string)
                      n266 = property on="Property Node" class="Str"(reference=w1712, "Value"=w1720) -> ()  [unwired: 1 in, 2 out]
                    }
                    n267 = call "Motors Stop.vi"("error in"=w1707, "Axis"=w1698, "VISA in"=w1708) -> ("error out"=w1705:errorcluster, "VISA out"=w1706:refnum<visa-resource-name>)
                  }
                }
              }
              frame #1 {
                n268 = property on="Property Node" class="Bool (strict)"(reference=w1730, "Value"=FALSE) -> ()  [unwired: 1 in, 2 out]
                n269 = property on="Property Node" class="Bool (strict)"(reference=w1731, "Value"=FALSE) -> ()  [unwired: 1 in, 2 out]
              }
            }
          }
        }
        n270 = Unbundle(w289) -> ("Jog-Mode"=w288:refnum<vi>, "y+?"=w276:refnum<vi>, "y-?"=w275:refnum<vi>, "Y Moving"=w278:refnum<vi>, "Delta Y (mm)"=w277:refnum<vi>, "Y Multiplier"=w285:refnum<vi>, "y+"=w284:refnum<vi>, "y-"=w283:refnum<vi>, "Y-Axis (mm)"=w281:refnum<vi>, "Status Y"=w282:refnum<vi>, "Y Speed (mm/s)"=w286:refnum<vi>)
        n271 = property on="Property Node" class="Bool (strict)"(reference=w288) -> ("Value"=w287:bool)  [unwired: 1 in, 2 out]
        n272 = property on="Property Node" class="Bool (strict)"(reference=w276) -> (reference out=w280:refnum<vi>, "Value"=w453:bool)  [unwired: 1 in, 1 out]
        n273 = property on="Property Node" class="Bool (strict)"(reference=w275) -> (reference out=w279:refnum<vi>, "Value"=w452:bool)  [unwired: 1 in, 1 out]
        n274 = Or(x=w453, y=w452) -> (x .or. y?=w479:bool)
        n275 = case shown="True" w479 {
          tunnel: w481 -> [w1521 w1538]
          tunnel: w480 -> [w1520 w1537]
          tunnel: w287 -> [_ w1539]
          tunnel: [w1521 w1536] -> w478
          tunnel: [w1520 w1535] -> w477
          tunnel: w452 -> [_ w1534]
          tunnel: w286 -> [_ w1531]
          tunnel: w285 -> [_ w1530]
          tunnel: w284 -> [_ w1529]
          tunnel: w283 -> [_ w1528]
          tunnel: w282 -> [_ w1527]
          tunnel: w281 -> [_ w1526]
          tunnel: w280 -> [_ w1525]
          tunnel: w279 -> [_ w1524]
          tunnel: w278 -> [_ w1523]
          tunnel: w277 -> [_ w1522]
          frame False {
          }
          frame True {
            n276 = flat-sequence {
              tunnel: w1539 -> [w1553]
              tunnel: w1538 -> [w1552]
              tunnel: w1537 -> [w1551]
              tunnel: w1534 -> [w1548]
              tunnel: [w1550] -> w1533
              tunnel: [w1549] -> w1532
              tunnel: w1531 -> [w1547]
              tunnel: w1530 -> [w1546]
              tunnel: w1529 -> [w1545]
              tunnel: w1528 -> [w1544]
              tunnel: w1527 -> [w1543]
              tunnel: w1526 -> [w1542]
              tunnel: w1523 -> [w1541]
              tunnel: w1522 -> [w1540]
              tunnel: [w1626] -> w1535
              tunnel: [w1627] -> w1536
              tunnel: w1533 -> [w1627]
              tunnel: w1532 -> [w1626]
              tunnel: w1525 -> [w1623]
              tunnel: w1524 -> [w1622]
              frame #0 {
                n277 = case shown="False" w1553 {
                  tunnel: w1552 -> [w1563 w1593]
                  tunnel: w1551 -> [w1562 w1596]
                  tunnel: [w1561 w1599] -> w1550
                  tunnel: [w1560 w1598] -> w1549
                  tunnel: w1548 -> [w1559 w1597]
                  tunnel: w1547 -> [_ w1588]
                  tunnel: w1546 -> [w1557 w1587]
                  tunnel: w1545 -> [_ w1586]
                  tunnel: w1544 -> [_ w1585]
                  tunnel: w1543 -> [_ w1584]
                  tunnel: w1542 -> [_ w1583]
                  tunnel: w1541 -> [w1556 _]
                  tunnel: w1540 -> [w1554 _]
                  frame False {
                    n278 = property on="Property Node" class="Bool (strict)"(reference=w1556) -> (reference out=w1555:refnum<vi>, "Value"=w1558:bool)  [unwired: 1 in, 1 out]
                    n279 = case shown="False" w1558 {
                      tunnel: w1563 -> [w1572 w1582]
                      tunnel: w1562 -> [w1576 w1581]
                      tunnel: [w1573 w1582] -> w1561
                      tunnel: [w1575 w1581] -> w1560
                      tunnel: w1559 -> [w1574 _]
                      tunnel: w1557 -> [w1567 _]
                      tunnel: w1555 -> [w1566 _]
                      tunnel: w1554 -> [w1565 _]
                      frame False {
                        n280 = property on="Property Node" class="Bool (strict)"(reference=w1566, "Value"=TRUE ("Y Moving")) -> ()  [unwired: 1 in, 2 out]
                        n281 = property on="Property Node" class="DigNum (strict)"(reference=w1565) -> ("Value"=w1564:dbl)  [unwired: 1 in, 2 out]
                        n282 = property on="Property Node" class="DigNum (strict)"(reference=w1567) -> ("Value"=w1569:u32)  [unwired: 1 in, 2 out]
                        n283 = case shown="True" w1574 {
                          tunnel: w1564 -> [w1577 w1579]
                          tunnel: [w1577 w1578] -> w1571
                          frame False {
                          }
                          frame True {
                            n284 = Multiply(x=w1579, y=-1.0) -> (x*y=w1578:dbl)
                          }
                        }
                        n285 = call "Motors Move Relative.vi"("Axis Multiplier"=w1569, "Axis"=2, "error in"=w1576, "VISA in"=w1572, "Distance (mm)"=w1571) -> ("error out"=w1575:errorcluster, "VISA out"=w1573:refnum<visa-resource-name>)  [unwired: 5 in]
                      }
                      frame True {
                      }
                    }
                  }
                  frame True {
                    w1590 = 2 ("Axis")
                    n286 = property on="Property Node" class="DigNum (strict)"(reference=w1587) -> ("Value"=w1591:u32)  [unwired: 1 in, 2 out]
                    n287 = property on="Property Node" class="DigNum (strict)"(reference=w1588) -> ("Value"=w1589:dbl)  [unwired: 1 in, 2 out]
                    n288 = case shown="True" w1597 {
                      tunnel: w1589 -> [w1618 w1620]
                      tunnel: [w1618 w1619] -> w1594
                      frame False {
                      }
                      frame True {
                        n289 = Multiply(x=w1620, y=-1.0) -> (x*y=w1619:dbl)
                      }
                    }
                    n290 = call "Motors Move Constant Velocity.vi"("Axis Multiplier"=w1591, "Axis"=w1590, "error in"=w1596, "VISA in"=w1593, "Speed (mm/s)"=w1594) -> ("error out"=w1595:errorcluster, "VISA out"=w1592:refnum<visa-resource-name>)  [unwired: 5 in]
                    n291 = while {
                      tunnel: w1592 -> [w1608]
                      tunnel: [w1607] -> w1601
                      tunnel: w1595 -> [w1610]
                      tunnel: [w1609] -> w1600
                      tunnel: w1591 -> [w1606]
                      tunnel: w1586 -> [w1605]
                      tunnel: w1585 -> [w1604]
                      tunnel: w1584 -> [w1603]
                      tunnel: w1583 -> [w1602]
                      stop <- w1617 continue-if-true
                      n292 = property on="Property Node" class="Bool (strict)"(reference=w1605) -> ("Value"=w1616:bool)  [unwired: 1 in, 2 out]
                      n293 = property on="Property Node" class="Bool (strict)"(reference=w1604) -> ("Value"=w1615:bool)  [unwired: 1 in, 2 out]
                      n294 = Or(x=w1616, y=w1615) -> (x .or. y?=w1617:bool)
                      n295 = call "Motors Status.vi"("error in"=w1610, "VISA in"=w1608, "Axis"=2, "Axis Multiplier"=w1606) -> ("error out"=w1609:errorcluster, "VISA out"=w1607:refnum<visa-resource-name>, "OS"=w1612:i32, "Actual Position (mm or deg)"=w1613:dbl)  [unwired: 3 in]
                      n296 = property on="Property Node" class="DigNum (strict)"(reference=w1602, "Value"=w1613) -> ()  [unwired: 1 in, 2 out]
                      n297 = call "Motors Decipher Status.vi"("OS"=w1612) -> ("Status"=w1611:string)
                      n298 = property on="Property Node" class="Str"(reference=w1603, "Value"=w1611) -> ()  [unwired: 1 in, 2 out]
                    }
                    n299 = call "Motors Stop.vi"("error in"=w1600, "Axis"=w1590, "VISA in"=w1601) -> ("error out"=w1598:errorcluster, "VISA out"=w1599:refnum<visa-resource-name>)
                  }
                }
              }
              frame #1 {
                n300 = property on="Property Node" class="Bool (strict)"(reference=w1623, "Value"=FALSE) -> ()  [unwired: 1 in, 2 out]
                n301 = property on="Property Node" class="Bool (strict)"(reference=w1622, "Value"=FALSE) -> ()  [unwired: 1 in, 2 out]
              }
            }
          }
        }
        n302 = Unbundle(w274) -> ("Jog-Mode"=w271:refnum<vi>, "z+?"=w273:refnum<vi>, "z-?"=w272:refnum<vi>, "Z Speed (mm/s)"=w266:refnum<vi>, "Delta Z (mm)"=w268:refnum<vi>, "Z Multiplier"=w267:refnum<vi>, "Z-Axis (mm)"=w263:refnum<vi>, "Status Z"=w262:refnum<vi>, "z+"=w265:refnum<vi>, "z-"=w264:refnum<vi>, "Z Moving"=w269:refnum<vi>)
        n303 = property on="Property Node" class="Bool (strict)"(reference=w273) -> (reference out=w415:refnum<vi>, "Value"=w450:bool)  [unwired: 1 in, 1 out]
        n304 = property on="Property Node" class="Bool (strict)"(reference=w272) -> (reference out=w416:refnum<vi>, "Value"=w451:bool)  [unwired: 1 in, 1 out]
        n305 = property on="Property Node" class="Bool (strict)"(reference=w271) -> ("Value"=w270:bool)  [unwired: 1 in, 2 out]
        n306 = Or(x=w450, y=w451) -> (x .or. y?=w476:bool)
        n307 = case shown="True" w476 {
          tunnel: w478 -> [w1409 w1427]
          tunnel: w477 -> [w1408 w1421]
          tunnel: w270 -> [_ w1428]
          tunnel: [w1409 w1426] -> w473
          tunnel: [w1408 w1425] -> w474
          tunnel: w451 -> [_ w1424]
          tunnel: w416 -> [_ w1420]
          tunnel: w416 -> [_ w1419]
          tunnel: w415 -> [_ w1418]
          tunnel: w269 -> [_ w1417]
          tunnel: w268 -> [_ w1416]
          tunnel: w267 -> [_ w1415]
          tunnel: w266 -> [_ w1414]
          tunnel: w265 -> [_ w1413]
          tunnel: w264 -> [_ w1412]
          tunnel: w263 -> [_ w1411]
          tunnel: w262 -> [_ w1410]
          frame False {
          }
          frame True {
            n308 = flat-sequence {
              tunnel: w1428 -> [w1443]
              tunnel: w1427 -> [w1442]
              tunnel: w1424 -> [w1439]
              tunnel: [w1441] -> w1423
              tunnel: [w1440] -> w1422
              tunnel: w1421 -> [w1438]
              tunnel: w1420 -> [w1437]
              tunnel: w1417 -> [w1436]
              tunnel: w1416 -> [w1435]
              tunnel: w1415 -> [w1434]
              tunnel: w1414 -> [w1433]
              tunnel: w1413 -> [w1432]
              tunnel: w1412 -> [w1431]
              tunnel: w1411 -> [w1430]
              tunnel: w1410 -> [w1429]
              tunnel: [w1518] -> w1425
              tunnel: [w1519] -> w1426
              tunnel: w1423 -> [w1519]
              tunnel: w1422 -> [w1518]
              tunnel: w1419 -> [w1515]
              tunnel: w1418 -> [w1514]
              frame #0 {
                n309 = case shown="True" w1443 {
                  tunnel: w1442 -> [w1453 w1485]
                  tunnel: w1438 -> [w1452 w1488]
                  tunnel: [w1451 w1491] -> w1441
                  tunnel: [w1450 w1490] -> w1440
                  tunnel: w1439 -> [w1449 w1480]
                  tunnel: w1438 -> [_ w1482]
                  tunnel: w1437 -> [_ w1479]
                  tunnel: w1436 -> [w1446 _]
                  tunnel: w1435 -> [w1445 _]
                  tunnel: w1434 -> [w1444 w1478]
                  tunnel: w1433 -> [_ w1477]
                  tunnel: w1432 -> [_ w1476]
                  tunnel: w1431 -> [_ w1475]
                  tunnel: w1430 -> [_ w1474]
                  tunnel: w1429 -> [_ w1473]
                  frame False {
                    n310 = property on="Property Node" class="Bool (strict)"(reference=w1446) -> (reference out=w1447:refnum<vi>, "Value"=w1448:bool)  [unwired: 1 in, 1 out]
                    n311 = case shown="False" w1448 {
                      tunnel: w1453 -> [w1459 w1472]
                      tunnel: w1452 -> [w1466 w1471]
                      tunnel: [w1460 w1472] -> w1451
                      tunnel: [w1465 w1471] -> w1450
                      tunnel: w1449 -> [w1464 _]
                      tunnel: w1447 -> [w1456 _]
                      tunnel: w1445 -> [w1455 _]
                      tunnel: w1444 -> [w1454 _]
                      frame False {
                        n312 = property on="Property Node" class="Bool (strict)"(reference=w1456, "Value"=TRUE ("Z Moving")) -> ()  [unwired: 1 in, 2 out]
                        n313 = property on="Property Node" class="DigNum (strict)"(reference=w1455) -> ("Value"=w1457:dbl)  [unwired: 1 in, 2 out]
                        n314 = property on="Property Node" class="DigNum (strict)"(reference=w1454) -> ("Value"=w1462:u32)  [unwired: 1 in, 2 out]
                        n315 = case shown="True" w1464 {
                          tunnel: w1457 -> [w1467 w1469]
                          tunnel: [w1467 w1468] -> w1461
                          frame False {
                          }
                          frame True {
                            n316 = Multiply(x=w1469, y=-1.0) -> (x*y=w1468:dbl)
                          }
                        }
                        n317 = call "Motors Move Relative.vi"("Axis Multiplier"=w1462, "Axis"=3, "error in"=w1466, "VISA in"=w1459, "Distance (mm)"=w1461) -> ("error out"=w1465:errorcluster, "VISA out"=w1460:refnum<visa-resource-name>)  [unwired: 5 in]
                      }
                      frame True {
                      }
                    }
                  }
                  frame True {
                    w1487 = 3 ("Axis")
                    n318 = property on="Property Node" class="DigNum (strict)"(reference=w1477, error in=w1482) -> ("Value"=w1481:dbl)  [unwired: 2 out]
                    n319 = property on="Property Node" class="DigNum (strict)"(reference=w1478) -> ("Value"=w1483:u32)  [unwired: 1 in, 2 out]
                    n320 = case shown="True" w1480 {
                      tunnel: w1481 -> [w1510 w1512]
                      tunnel: [w1510 w1511] -> w1486
                      frame False {
                      }
                      frame True {
                        n321 = Multiply(x=w1512, y=-1.0) -> (x*y=w1511:dbl)
                      }
                    }
                    n322 = call "Motors Move Constant Velocity.vi"("Axis Multiplier"=w1483, "Axis"=w1487, "error in"=w1488, "VISA in"=w1485, "Speed (mm/s)"=w1486) -> ("error out"=w1489:errorcluster, "VISA out"=w1484:refnum<visa-resource-name>)  [unwired: 5 in]
                    n323 = while {
                      tunnel: w1484 -> [w1500]
                      tunnel: [w1499] -> w1493
                      tunnel: w1489 -> [w1502]
                      tunnel: [w1501] -> w1492
                      tunnel: w1483 -> [w1498]
                      tunnel: w1479 -> [_]
                      tunnel: w1476 -> [w1497]
                      tunnel: w1475 -> [w1496]
                      tunnel: w1474 -> [w1495]
                      tunnel: w1473 -> [w1494]
                      stop <- w1509 continue-if-true
                      n324 = property on="Property Node" class="Bool (strict)"(reference=w1497) -> ("Value"=w1508:bool)  [unwired: 1 in, 2 out]
                      n325 = property on="Property Node" class="Bool (strict)"(reference=w1496) -> ("Value"=w1507:bool)  [unwired: 1 in, 2 out]
                      n326 = Or(x=w1508, y=w1507) -> (x .or. y?=w1509:bool)
                      n327 = call "Motors Status.vi"("error in"=w1502, "VISA in"=w1500, "Axis"=3, "Axis Multiplier"=w1498) -> ("error out"=w1501:errorcluster, "VISA out"=w1499:refnum<visa-resource-name>, "OS"=w1504:i32, "Actual Position (mm or deg)"=w1505:dbl)  [unwired: 3 in]
                      n328 = property on="Property Node" class="DigNum (strict)"(reference=w1495, "Value"=w1505) -> ()  [unwired: 1 in, 2 out]
                      n329 = call "Motors Decipher Status.vi"("OS"=w1504) -> ("Status"=w1503:string)
                      n330 = property on="Property Node" class="Str"(reference=w1494, "Value"=w1503) -> ()  [unwired: 1 in, 2 out]
                    }
                    n331 = call "Motors Stop.vi"("error in"=w1492, "Axis"=w1487, "VISA in"=w1493) -> ("error out"=w1490:errorcluster, "VISA out"=w1491:refnum<visa-resource-name>)
                  }
                }
              }
              frame #1 {
                n332 = property on="Property Node" class="Bool (strict)"(reference=w1514, "Value"=FALSE) -> ()  [unwired: 1 in, 2 out]
                n333 = property on="Property Node" class="Bool (strict)"(reference=w1515, "Value"=FALSE) -> ()  [unwired: 1 in, 2 out]
              }
            }
          }
        }
        n334 = Unbundle(w261) -> ("Jog-Mode"=w260:refnum<vi>, "theta+?"=w259:refnum<vi>, "theta-?"=w258:refnum<vi>, "Theta Speed (deg/s)"=w254:refnum<vi>, "Delta Theta (deg)"=w248:refnum<vi>, "Theta Multiplier"=w255:refnum<vi>, "Theta (deg)"=w251:refnum<vi>, "Status Theta"=w250:refnum<vi>, "theta+"=w253:refnum<vi>, "theta-"=w252:refnum<vi>, "Theta Moving"=w249:refnum<vi>)
        n335 = property on="Property Node" class="Bool (strict)"(reference=w259) -> (reference out=w256:refnum<vi>, "Value"=w449:bool)  [unwired: 1 in, 1 out]
        n336 = property on="Property Node" class="Bool (strict)"(reference=w258) -> (reference out=w257:refnum<vi>, "Value"=w448:bool)  [unwired: 1 in, 1 out]
        n337 = property on="Property Node" class="Bool (strict)"(reference=w260) -> ("Value"=w299:bool)  [unwired: 1 in, 2 out]
        n338 = Or(x=w449, y=w448) -> (x .or. y?=w475:bool)
        n339 = case shown="True" w475 {
          tunnel: w473 -> [w1301 w1318]
          tunnel: w474 -> [w1300 w1317]
          tunnel: w299 -> [_ w1319]
          tunnel: [w1301 w1316] -> w472
          tunnel: [w1300 w1315] -> w465
          tunnel: w448 -> [_ w1314]
          tunnel: w257 -> [_ w1311]
          tunnel: w256 -> [_ w1310]
          tunnel: w255 -> [_ w1309]
          tunnel: w254 -> [_ w1308]
          tunnel: w253 -> [_ w1307]
          tunnel: w252 -> [_ w1306]
          tunnel: w251 -> [_ w1305]
          tunnel: w250 -> [_ w1304]
          tunnel: w249 -> [_ w1303]
          tunnel: w248 -> [_ w1302]
          frame False {
          }
          frame True {
            n340 = flat-sequence {
              tunnel: w1319 -> [w1333]
              tunnel: w1318 -> [w1332]
              tunnel: w1317 -> [w1331]
              tunnel: w1314 -> [w1328]
              tunnel: [w1330] -> w1313
              tunnel: [w1329] -> w1312
              tunnel: w1309 -> [w1327]
              tunnel: w1308 -> [w1326]
              tunnel: w1307 -> [w1325]
              tunnel: w1306 -> [w1324]
              tunnel: w1305 -> [w1323]
              tunnel: w1304 -> [w1322]
              tunnel: w1303 -> [w1321]
              tunnel: w1302 -> [w1320]
              tunnel: [w1406] -> w1315
              tunnel: [w1407] -> w1316
              tunnel: w1313 -> [w1407]
              tunnel: w1312 -> [w1406]
              tunnel: w1311 -> [w1403]
              tunnel: w1310 -> [w1402]
              frame #0 {
                n341 = case shown="False" w1333 {
                  tunnel: w1332 -> [w1343 w1374]
                  tunnel: w1331 -> [w1342 w1375]
                  tunnel: [w1341 w1379] -> w1330
                  tunnel: [w1340 w1378] -> w1329
                  tunnel: w1328 -> [w1339 w1377]
                  tunnel: w1327 -> [w1337 w1369]
                  tunnel: w1326 -> [_ w1367]
                  tunnel: w1325 -> [_ w1366]
                  tunnel: w1324 -> [_ w1365]
                  tunnel: w1323 -> [_ w1364]
                  tunnel: w1322 -> [_ w1363]
                  tunnel: w1321 -> [w1336 _]
                  tunnel: w1320 -> [w1334 _]
                  frame False {
                    n342 = property on="Property Node" class="Bool (strict)"(reference=w1336) -> (reference out=w1335:refnum<vi>, "Value"=w1338:bool)  [unwired: 1 in, 1 out]
                    n343 = case shown="False" w1338 {
                      tunnel: w1343 -> [w1350 w1362]
                      tunnel: w1342 -> [w1356 w1361]
                      tunnel: [w1351 w1362] -> w1341
                      tunnel: [w1355 w1361] -> w1340
                      tunnel: w1339 -> [w1354 _]
                      tunnel: w1337 -> [w1347 _]
                      tunnel: w1335 -> [w1346 _]
                      tunnel: w1334 -> [w1345 _]
                      frame False {
                        n344 = property on="Property Node" class="Bool (strict)"(reference=w1346, "Value"=TRUE ("Theta Moving")) -> ()  [unwired: 1 in, 2 out]
                        n345 = property on="Property Node" class="DigNum (strict)"(reference=w1345) -> ("Value"=w1344:dbl)  [unwired: 1 in, 2 out]
                        n346 = property on="Property Node" class="DigNum (strict)"(reference=w1347) -> ("Value"=w1353:u32)  [unwired: 1 in, 2 out]
                        n347 = case shown="True" w1354 {
                          tunnel: w1344 -> [w1357 w1359]
                          tunnel: [w1357 w1358] -> w1349
                          frame False {
                          }
                          frame True {
                            n348 = Multiply(x=w1359, y=-1.0) -> (x*y=w1358:dbl)
                          }
                        }
                        n349 = call "Motors Move Relative.vi"("Axis Multiplier"=w1353, "Axis"=4, "error in"=w1356, "VISA in"=w1350, "Distance (mm)"=w1349) -> ("error out"=w1355:errorcluster, "VISA out"=w1351:refnum<visa-resource-name>)  [unwired: 5 in]
                      }
                      frame True {
                      }
                    }
                  }
                  frame True {
                    w1372 = 4 ("Axis")
                    n350 = property on="Property Node" class="DigNum (strict)"(reference=w1367) -> ("Value"=w1368:dbl)  [unwired: 1 in, 2 out]
                    n351 = property on="Property Node" class="DigNum (strict)"(reference=w1369) -> ("Value"=w1371:u32)  [unwired: 1 in, 2 out]
                    n352 = case shown="True" w1377 {
                      tunnel: w1368 -> [w1398 w1400]
                      tunnel: [w1398 w1399] -> w1370
                      frame False {
                      }
                      frame True {
                        n353 = Multiply(x=w1400, y=-1.0) -> (x*y=w1399:dbl)
                      }
                    }
                    n354 = call "Motors Move Constant Velocity.vi"("Axis Multiplier"=w1371, "Axis"=w1372, "error in"=w1375, "VISA in"=w1374, "Speed (mm/s)"=w1370) -> ("error out"=w1376:errorcluster, "VISA out"=w1373:refnum<visa-resource-name>)  [unwired: 5 in]
                    n355 = while {
                      tunnel: w1373 -> [w1388]
                      tunnel: [w1387] -> w1381
                      tunnel: w1376 -> [w1390]
                      tunnel: [w1389] -> w1380
                      tunnel: w1371 -> [w1386]
                      tunnel: w1366 -> [w1385]
                      tunnel: w1365 -> [w1384]
                      tunnel: w1364 -> [w1383]
                      tunnel: w1363 -> [w1382]
                      stop <- w1397 continue-if-true
                      n356 = property on="Property Node" class="Bool (strict)"(reference=w1385) -> ("Value"=w1396:bool)  [unwired: 1 in, 2 out]
                      n357 = property on="Property Node" class="Bool (strict)"(reference=w1384) -> ("Value"=w1395:bool)  [unwired: 1 in, 2 out]
                      n358 = Or(x=w1396, y=w1395) -> (x .or. y?=w1397:bool)
                      n359 = call "Motors Status.vi"("error in"=w1390, "VISA in"=w1388, "Axis"=4, "Axis Multiplier"=w1386) -> ("error out"=w1389:errorcluster, "VISA out"=w1387:refnum<visa-resource-name>, "OS"=w1392:i32, "Actual Position (mm or deg)"=w1393:dbl)  [unwired: 3 in]
                      n360 = property on="Property Node" class="DigNum (strict)"(reference=w1383, "Value"=w1393) -> ()  [unwired: 1 in, 2 out]
                      n361 = call "Motors Decipher Status.vi"("OS"=w1392) -> ("Status"=w1391:string)
                      n362 = property on="Property Node" class="Str"(reference=w1382, "Value"=w1391) -> ()  [unwired: 1 in, 2 out]
                    }
                    n363 = call "Motors Stop.vi"("error in"=w1380, "Axis"=w1372, "VISA in"=w1381) -> ("error out"=w1378:errorcluster, "VISA out"=w1379:refnum<visa-resource-name>)
                  }
                }
              }
              frame #1 {
                n364 = property on="Property Node" class="Bool (strict)"(reference=w1402, "Value"=FALSE) -> ()  [unwired: 1 in, 2 out]
                n365 = property on="Property Node" class="Bool (strict)"(reference=w1403, "Value"=FALSE) -> ()  [unwired: 1 in, 2 out]
              }
            }
          }
        }
        n366 = Unbundle(w247) -> ("X Set Slew Speed?"=w245:refnum<vi>, "(mm/s)"=w239:refnum<vi>, "Y Set Slew Speed?"=w235:refnum<vi>, "(mm/s)"=w238:refnum<vi>, "Z Set Slew Speed?"=w233:refnum<vi>, "(mm/s)"=w237:refnum<vi>, "Theta Set Slew Speed?"=w231:refnum<vi>, "(degrees/s)"=w236:refnum<vi>, "Need to Update Motor Parameters"=w244:refnum<vi>, "X Multiplier"=w243:refnum<vi>, "Y Multiplier"=w242:refnum<vi>, "Z Multiplier"=w241:refnum<vi>, "Theta Multiplier"=w240:refnum<vi>)
        n367 = property on="Property Node" class="Bool (strict)"(reference=w245) -> (reference out=w229:refnum<vi>, "Value"=w246:bool)  [unwired: 1 in, 1 out]
        n368 = case shown="True" w246 {
          tunnel: [w1286 w1294] -> w469
          tunnel: w472 -> [w1286 w1295]
          tunnel: [w1285 w1298] -> w466
          tunnel: w465 -> [w1285 w1299]
          tunnel: w244 -> [_ w1292]
          tunnel: w243 -> [_ w1291]
          tunnel: w239 -> [_ w1290]
          tunnel: w229 -> [_ w1287]
          frame False {
          }
          frame True {
            n369 = property on="Property Node" class="DigNum (strict)"(reference=w1290) -> ("Value"=w1289:dbl)  [unwired: 1 in, 2 out]
            n370 = property on="Property Node" class="DigNum (strict)"(reference=w1291) -> ("Value"=w1293:u32)  [unwired: 1 in, 2 out]
            n371 = property on="Property Node" class="Bool (strict)"(reference=w1287, "Value"=FALSE) -> ()  [unwired: 1 in, 2 out]
            n372 = property on="Property Node" class="Bool (strict)"(reference=w1292, "Value"=TRUE ("Need to Update Motor Parameters")) -> ()  [unwired: 1 in, 2 out]
            n373 = call "Motors Move Speed.vi"("Speed (mm or degree/sec)"=w1289, "error in"=w1299, "VISA in"=w1295, "Axis"=u32 1, "Axis Multiplier"=w1293) -> ("error out"=w1298:errorcluster, "VISA out"=w1294:refnum<visa-resource-name>)  [unwired: 5 in]
          }
        }
        n374 = property on="Property Node" class="Bool (strict)"(reference=w235) -> (reference out=w228:refnum<vi>, "Value"=w234:bool)  [unwired: 1 in, 1 out]
        n375 = case shown="True" w234 {
          tunnel: [w1271 w1280] -> w470
          tunnel: w469 -> [w1271 w1278]
          tunnel: [w1270 w1283] -> w467
          tunnel: w466 -> [w1270 w1284]
          tunnel: w244 -> [_ w1277]
          tunnel: w242 -> [_ w1276]
          tunnel: w238 -> [_ w1275]
          tunnel: w228 -> [_ w1272]
          frame False {
          }
          frame True {
            n376 = property on="Property Node" class="DigNum (strict)"(reference=w1275) -> ("Value"=w1274:dbl)  [unwired: 1 in, 2 out]
            n377 = property on="Property Node" class="DigNum (strict)"(reference=w1276) -> ("Value"=w1279:u32)  [unwired: 1 in, 2 out]
            n378 = property on="Property Node" class="Bool (strict)"(reference=w1272, "Value"=FALSE) -> ()  [unwired: 1 in, 2 out]
            n379 = property on="Property Node" class="Bool (strict)"(reference=w1277, "Value"=TRUE ("Need to Update Motor Parameters")) -> ()  [unwired: 1 in, 2 out]
            n380 = call "Motors Move Speed.vi"("Speed (mm or degree/sec)"=w1274, "error in"=w1284, "VISA in"=w1278, "Axis"=u32 2, "Axis Multiplier"=w1279) -> ("error out"=w1283:errorcluster, "VISA out"=w1280:refnum<visa-resource-name>)  [unwired: 5 in]
          }
        }
        n381 = property on="Property Node" class="Bool (strict)"(reference=w233) -> (reference out=w227:refnum<vi>, "Value"=w232:bool)  [unwired: 1 in, 1 out]
        n382 = case shown="True" w232 {
          tunnel: [w1256 w1265] -> w471
          tunnel: w470 -> [w1256 w1264]
          tunnel: [w1255 w1268] -> w468
          tunnel: w467 -> [w1255 w1269]
          tunnel: w244 -> [_ w1262]
          tunnel: w241 -> [_ w1261]
          tunnel: w237 -> [_ w1260]
          tunnel: w227 -> [_ w1257]
          frame False {
          }
          frame True {
            n383 = property on="Property Node" class="DigNum (strict)"(reference=w1260) -> ("Value"=w1259:dbl)  [unwired: 1 in, 2 out]
            n384 = property on="Property Node" class="DigNum (strict)"(reference=w1261) -> ("Value"=w1263:u32)  [unwired: 1 in, 2 out]
            n385 = property on="Property Node" class="Bool (strict)"(reference=w1257, "Value"=FALSE) -> ()  [unwired: 1 in, 2 out]
            n386 = property on="Property Node" class="Bool (strict)"(reference=w1262, "Value"=TRUE ("Need to Update Motor Parameters")) -> ()  [unwired: 1 in, 2 out]
            n387 = call "Motors Move Speed.vi"("Speed (mm or degree/sec)"=w1259, "error in"=w1269, "VISA in"=w1264, "Axis"=u32 3, "Axis Multiplier"=w1263) -> ("error out"=w1268:errorcluster, "VISA out"=w1265:refnum<visa-resource-name>)  [unwired: 5 in]
          }
        }
        n388 = property on="Property Node" class="Bool (strict)"(reference=w231) -> (reference out=w226:refnum<vi>, "Value"=w230:bool)  [unwired: 1 in, 1 out]
        n389 = case shown="True" w230 {
          tunnel: [w1241 w1250] -> w463
          tunnel: w471 -> [w1241 w1249]
          tunnel: [w1240 w1251] -> w464
          tunnel: w468 -> [w1240 w1254]
          tunnel: w244 -> [_ w1247]
          tunnel: w240 -> [_ w1246]
          tunnel: w236 -> [_ w1245]
          tunnel: w226 -> [_ w1242]
          frame False {
          }
          frame True {
            n390 = property on="Property Node" class="DigNum (strict)"(reference=w1245) -> ("Value"=w1244:dbl)  [unwired: 1 in, 2 out]
            n391 = property on="Property Node" class="DigNum (strict)"(reference=w1246) -> ("Value"=w1248:u32)  [unwired: 1 in, 2 out]
            n392 = property on="Property Node" class="Bool (strict)"(reference=w1247, "Value"=TRUE ("Need to Update Motor Parameters")) -> ()  [unwired: 1 in, 2 out]
            n393 = property on="Property Node" class="Bool (strict)"(reference=w1242, "Value"=FALSE) -> ()  [unwired: 1 in, 2 out]
            n394 = call "Motors Move Speed.vi"("Speed (mm or degree/sec)"=w1244, "error in"=w1254, "VISA in"=w1249, "Axis"=u32 4, "Axis Multiplier"=w1248) -> ("error out"=w1251:errorcluster, "VISA out"=w1250:refnum<visa-resource-name>)  [unwired: 5 in]
          }
        }
        n395 = Quotient & Remainder(x=w440, y=4) -> (x-y*floor(x/y)=w461:i32)  [unwired: 1 out]
        n396 = Unbundle(w225) -> ("Status X"=w224:refnum<vi>, "X-Axis (mm)"=w223:refnum<vi>, "X Multiplier"=w222:refnum<vi>, "X Moving"=w221:refnum<vi>, "Status Y"=w220:refnum<vi>, "Y-Axis (mm)"=w219:refnum<vi>, "Y Multiplier"=w218:refnum<vi>, "Y Moving"=w217:refnum<vi>, "Status Z"=w216:refnum<vi>, "Z-Axis (mm)"=w215:refnum<vi>, "Z Multiplier"=w214:refnum<vi>, "Z Moving"=w213:refnum<vi>, "Status Theta"=w212:refnum<vi>, "Theta (deg)"=w211:refnum<vi>, "Theta Multiplier"=w210:refnum<vi>, "Theta Moving"=w209:refnum<vi>)
        n397 = case shown="0, Default" w461 {
          tunnel: w464 -> [w1056 w1074 w1091 w1110]
          tunnel: w463 -> [w1057 w1075 w1093 w1111]
          tunnel: [w1055 w1072 w1090 w1109] -> w459
          tunnel: [w1054 w1073 w1092 w1108] -> w458
          tunnel: w224 -> [w1052 _ _ _]
          tunnel: w223 -> [w1051 _ _ _]
          tunnel: w222 -> [w1050 _ _ _]
          tunnel: w221 -> [w1049 _ _ _]
          tunnel: w220 -> [_ w1070 _ _]
          tunnel: w219 -> [_ w1069 _ _]
          tunnel: w218 -> [_ w1068 _ _]
          tunnel: w217 -> [_ w1067 _ _]
          tunnel: w216 -> [_ _ w1088 _]
          tunnel: w215 -> [_ _ w1087 _]
          tunnel: w214 -> [_ _ w1086 _]
          tunnel: w213 -> [_ _ w1085 _]
          tunnel: w212 -> [_ _ _ w1106]
          tunnel: w211 -> [_ _ _ w1105]
          tunnel: w210 -> [_ _ _ w1104]
          tunnel: w209 -> [_ _ _ w1103]
          frame 0, Default {
            n398 = property on="Property Node" class="DigNum (strict)"(reference=w1050) -> ("Value"=w1053:u32)  [unwired: 1 in, 2 out]
            n399 = call "Motors Status.vi"("error in"=w1056, "VISA in"=w1057, "Axis"=1, "Axis Multiplier"=w1053) -> ("error out"=w1055:errorcluster, "VISA out"=w1054:refnum<visa-resource-name>, "OS"=w1063:i32, "Actual Position (mm or deg)"=w1058:dbl)  [unwired: 3 in]
            n400 = property on="Property Node" class="DigNum (strict)"(reference=w1051, "Value"=w1058) -> ()  [unwired: 1 in, 2 out]
            n401 = call "Motors Decipher Status.vi"("OS"=w1063) -> ("Status"=w1062:string)
            n402 = property on="Property Node" class="Str"(reference=w1052, "Value"=w1062) -> ()  [unwired: 1 in, 2 out]
            n403 = Equal?(x=w1062, y="Idle") -> (x = y?=w1060:bool)
            n404 = case shown="False" w1060 {
              tunnel: [TRUE FALSE] -> w1059
              frame False {
              }
              frame True {
              }
            }
            n405 = property on="Property Node" class="Bool (strict)"(reference=w1049, "Value"=w1059) -> ()  [unwired: 1 in, 2 out]
          }
          frame 1 {
            n406 = property on="Property Node" class="DigNum (strict)"(reference=w1068) -> ("Value"=w1071:u32)  [unwired: 1 in, 2 out]
            n407 = call "Motors Status.vi"("error in"=w1074, "VISA in"=w1075, "Axis"=2, "Axis Multiplier"=w1071) -> ("error out"=w1072:errorcluster, "VISA out"=w1073:refnum<visa-resource-name>, "OS"=w1080:i32, "Actual Position (mm or deg)"=w1081:dbl)  [unwired: 3 in]
            n408 = property on="Property Node" class="DigNum (strict)"(reference=w1069, "Value"=w1081) -> ()  [unwired: 1 in, 2 out]
            n409 = call "Motors Decipher Status.vi"("OS"=w1080) -> ("Status"=w1078:string)
            n410 = property on="Property Node" class="Str"(reference=w1070, "Value"=w1078) -> ()  [unwired: 1 in, 2 out]
            n411 = Equal?(x=w1078, y="Idle") -> (x = y?=w1077:bool)
            n412 = case shown="False" w1077 {
              tunnel: [TRUE FALSE] -> w1076
              frame False {
              }
              frame True {
              }
            }
            n413 = property on="Property Node" class="Bool (strict)"(reference=w1067, "Value"=w1076) -> ()  [unwired: 1 in, 2 out]
          }
          frame 2 {
            n414 = property on="Property Node" class="DigNum (strict)"(reference=w1086) -> ("Value"=w1089:u32)  [unwired: 1 in, 2 out]
            n415 = call "Motors Status.vi"("error in"=w1091, "VISA in"=w1093, "Axis"=3, "Axis Multiplier"=w1089) -> ("error out"=w1090:errorcluster, "VISA out"=w1092:refnum<visa-resource-name>, "OS"=w1098:i32, "Actual Position (mm or deg)"=w1099:dbl)  [unwired: 3 in]
            n416 = property on="Property Node" class="DigNum (strict)"(reference=w1087, "Value"=w1099) -> ()  [unwired: 1 in, 2 out]
            n417 = call "Motors Decipher Status.vi"("OS"=w1098) -> ("Status"=w1096:string)
            n418 = property on="Property Node" class="Str"(reference=w1088, "Value"=w1096) -> ()  [unwired: 1 in, 2 out]
            n419 = Equal?(x=w1096, y="Idle") -> (x = y?=w1095:bool)
            n420 = case shown="False" w1095 {
              tunnel: [TRUE FALSE] -> w1094
              frame False {
              }
              frame True {
              }
            }
            n421 = property on="Property Node" class="Bool (strict)"(reference=w1085, "Value"=w1094) -> ()  [unwired: 1 in, 2 out]
          }
          frame 3 {
            n422 = property on="Property Node" class="DigNum (strict)"(reference=w1104) -> ("Value"=w1107:u32)  [unwired: 1 in, 2 out]
            n423 = call "Motors Status.vi"("error in"=w1110, "VISA in"=w1111, "Axis"=4, "Axis Multiplier"=w1107) -> ("error out"=w1109:errorcluster, "VISA out"=w1108:refnum<visa-resource-name>, "OS"=w1116:i32, "Actual Position (mm or deg)"=w1117:dbl)  [unwired: 3 in]
            n424 = property on="Property Node" class="DigNum (strict)"(reference=w1105, "Value"=w1117) -> ()  [unwired: 1 in, 2 out]
            n425 = call "Motors Decipher Status.vi"("OS"=w1116) -> ("Status"=w1114:string)
            n426 = property on="Property Node" class="Str"(reference=w1106, "Value"=w1114) -> ()  [unwired: 1 in, 2 out]
            n427 = Equal?(x=w1114, y="Idle") -> (x = y?=w1113:bool)
            n428 = case shown="True" w1113 {
              tunnel: [TRUE FALSE] -> w1112
              frame False {
              }
              frame True {
              }
            }
            n429 = property on="Property Node" class="Bool (strict)"(reference=w1103, "Value"=w1112) -> ()  [unwired: 1 in, 2 out]
          }
        }
        n430 = Unbundle(w208) -> ("Go To Saved Position?"=w206:refnum<vi>, "Defined Positions"=w204:refnum<vi>, "X Multiplier"=w202:refnum<vi>, "Y Multiplier"=w201:refnum<vi>, "Z Multiplier"=w200:refnum<vi>, "Theta Multiplier"=w199:refnum<vi>, "Saved Positions"=w203:refnum<vi>)
        n431 = property on="Property Node" class="Bool (strict)"(reference=w206) -> (reference out=w205:refnum<vi>, "Value"=w207:bool)  [unwired: 1 in, 1 out]
        n432 = case shown="True" w207 {
          tunnel: w459 -> [w1010 w1021]
          tunnel: w458 -> [w1009 w1027]
          tunnel: [w1010 w1040] -> w457
          tunnel: [w1009 w1039] -> w456
          tunnel: w205 -> [_ w1018]
          tunnel: w204 -> [_ w1017]
          tunnel: w203 -> [_ w1015]
          tunnel: w202 -> [_ w1014]
          tunnel: w201 -> [_ w1013]
          tunnel: w200 -> [_ w1012]
          tunnel: w199 -> [_ w1011]
          frame False {
          }
          frame True {
            w1037 = 4 ("index (row)")
            w1035 = 3 ("index (row)")
            w1032 = 2 ("index (row)")
            w1029 = 1 ("index (row)")
            n433 = property on="Property Node" class="DigNum (strict)"(reference=w1011) -> ("Value"=w1023:u32)  [unwired: 1 in, 2 out]
            n434 = property on="Property Node" class="DigNum (strict)"(reference=w1012) -> ("Value"=w1024:u32)  [unwired: 1 in, 2 out]
            n435 = property on="Property Node" class="DigNum (strict)"(reference=w1013) -> ("Value"=w1025:u32)  [unwired: 1 in, 2 out]
            n436 = property on="Property Node" class="DigNum (strict)"(reference=w1014) -> ("Value"=w1026:u32)  [unwired: 1 in, 2 out]
            n437 = property on="Property Node" class="LstBox (strict)"(reference=w1017) -> ("Value"=w1016:i32)  [unwired: 1 in, 2 out]
            n438 = property on="Property Node" class="Bool (strict)"(reference=w1018, "Value"=FALSE) -> ()  [unwired: 1 in, 2 out]
            n439 = property on="Property Node" class="Path"(reference=w1015) -> ("Value"=w1022:path)  [unwired: 1 in, 2 out]
            n440 = call "Motors Position Load.vi"("error in"=w1021, "file path"=w1022) -> ("error out"=w1020:errorcluster, "Positions"=w1043:string[][])
            n441 = Index Array(array=w1043, index (row)=w1037, index (col)=w1016) -> (element=w1044:string)
            n442 = Index Array(array=w1043, index (row)=w1035, index (col)=w1016) -> (element=w1045:string)
            n443 = Index Array(array=w1043, index (row)=w1032, index (col)=w1016) -> (element=w1047:string)
            n444 = Index Array(array=w1043, index (row)=w1029, index (col)=w1016) -> (element=w1048:string)
            n445 = Fract/Exp String To Number(string=w1044) -> (number=w1038:dbl)  [unwired: 3 in, 1 out]
            n446 = Fract/Exp String To Number(string=w1045) -> (number=w1034:dbl)  [unwired: 3 in, 1 out]
            n447 = Fract/Exp String To Number(string=w1047) -> (number=w1031:dbl)  [unwired: 3 in, 1 out]
            n448 = Fract/Exp String To Number(string=w1048) -> (number=w1028:dbl)  [unwired: 3 in, 1 out]
            n449 = call "Motors Move Absolute.vi"("Axis Multiplier"=w1026, "Axis"=w1029, "error in"=w1020, "VISA in"=w1027, "Position (mm or degree)"=w1028) -> ("error out"=w1046:errorcluster, "VISA out"=w1030:refnum<visa-resource-name>)  [unwired: 5 in]
            n450 = call "Motors Move Absolute.vi"("Axis Multiplier"=w1025, "Axis"=w1032, "error in"=w1046, "VISA in"=w1030, "Position (mm or degree)"=w1031) -> ("error out"=w1042:errorcluster, "VISA out"=w1033:refnum<visa-resource-name>)  [unwired: 5 in]
            n451 = call "Motors Move Absolute.vi"("Axis Multiplier"=w1024, "Axis"=w1035, "error in"=w1042, "VISA in"=w1033, "Position (mm or degree)"=w1034) -> ("error out"=w1041:errorcluster, "VISA out"=w1036:refnum<visa-resource-name>)  [unwired: 5 in]
            n452 = call "Motors Move Absolute.vi"("Axis Multiplier"=w1023, "Axis"=w1037, "error in"=w1041, "VISA in"=w1036, "Position (mm or degree)"=w1038) -> ("error out"=w1040:errorcluster, "VISA out"=w1039:refnum<visa-resource-name>)  [unwired: 5 in]
          }
        }
        n453 = Unbundle(w197) -> ("Need to Update Motor Parameters"=w196:refnum<vi>, "X Jogger Normal Speed"=w193:refnum<vi>, "X Jogger Fast Speed"=w192:refnum<vi>, "X Slew Speed (mm or degree/s)"=w194:refnum<vi>, "X-Axis (mm)"=w191:refnum<vi>, "Status X"=w190:refnum<vi>, "X Moving"=w189:refnum<vi>)
        n454 = property on="Property Node" class="Bool (strict)"(reference=w196) -> (reference out=w195:refnum<vi>, "Value"=w462:bool)  [unwired: 1 in, 1 out]
        n455 = Unbundle(w188) -> ("Y Slew Speed (mm or degree/s)"=w187:refnum<vi>, "Y Jogger Normal Speed"=w186:refnum<vi>, "Y Jogger Fast Speed"=w185:refnum<vi>, "Y-Axis (mm)"=w184:refnum<vi>, "Status Y"=w183:refnum<vi>, "Y Moving"=w182:refnum<vi>)
        n456 = Unbundle(w181) -> ("Z Slew Speed (mm or degree/s)"=w180:refnum<vi>, "Z Jogger Normal Speed"=w179:refnum<vi>, "Z Jogger Fast Speed"=w178:refnum<vi>, "Z-Axis (mm)"=w177:refnum<vi>, "Status Z"=w176:refnum<vi>, "Z Moving"=w175:refnum<vi>)
        n457 = Unbundle(w174) -> ("Theta Slew Speed (mm or degree/s)"=w173:refnum<vi>, "Theta Jogger Normal Speed"=w172:refnum<vi>, "Theta Jogger Fast Speed"=w171:refnum<vi>, "Theta (deg)"=w170:refnum<vi>, "Status Theta"=w169:refnum<vi>, "Theta Moving"=w168:refnum<vi>)
        n458 = case shown="True" w462 {
          tunnel: w457 -> [w1122 w1153]
          tunnel: w456 -> [w1121 w1154]
          tunnel: [w1121 w1152] -> w167
          tunnel: [w1122 w1151] -> w447
          tunnel: w198 -> [_ w1150]
          tunnel: w195 -> [_ w1149]
          tunnel: w194 -> [_ w1148]
          tunnel: w193 -> [_ w1147]
          tunnel: w192 -> [_ w1146]
          tunnel: w191 -> [_ w1145]
          tunnel: w190 -> [_ w1144]
          tunnel: w189 -> [_ w1143]
          tunnel: w187 -> [_ w1142]
          tunnel: w186 -> [_ w1141]
          tunnel: w185 -> [_ w1140]
          tunnel: w184 -> [_ w1139]
          tunnel: w183 -> [_ w1138]
          tunnel: w182 -> [_ w1137]
          tunnel: w180 -> [_ w1136]
          tunnel: w179 -> [_ w1135]
          tunnel: w178 -> [_ w1134]
          tunnel: w177 -> [_ w1133]
          tunnel: w176 -> [_ w1132]
          tunnel: w175 -> [_ w1131]
          tunnel: w173 -> [_ w1130]
          tunnel: w172 -> [_ w1129]
          tunnel: w171 -> [_ w1128]
          tunnel: w170 -> [_ w1127]
          tunnel: w169 -> [_ w1126]
          tunnel: w168 -> [_ w1125]
          frame False {
          }
          frame True {
            n459 = flat-sequence {
              tunnel: w1150 -> [w1157]
              tunnel: [w1156] -> w1124
              tunnel: w1154 -> [w1192]
              tunnel: w1153 -> [w1191]
              tunnel: [w1190] -> w1152
              tunnel: [w1189] -> w1151
              tunnel: w1148 -> [w1182]
              tunnel: w1147 -> [w1187]
              tunnel: w1146 -> [w1186]
              tunnel: w1145 -> [w1185]
              tunnel: w1144 -> [w1184]
              tunnel: w1143 -> [w1183]
              tunnel: w1142 -> [w1169]
              tunnel: w1141 -> [w1180]
              tunnel: w1140 -> [w1179]
              tunnel: w1139 -> [w1178]
              tunnel: w1138 -> [w1177]
              tunnel: w1137 -> [w1176]
              tunnel: w1136 -> [w1167]
              tunnel: w1135 -> [w1175]
              tunnel: w1134 -> [w1174]
              tunnel: w1133 -> [w1173]
              tunnel: w1132 -> [w1172]
              tunnel: w1131 -> [w1171]
              tunnel: w1130 -> [w1160]
              tunnel: w1129 -> [w1166]
              tunnel: w1128 -> [w1165]
              tunnel: w1127 -> [w1164]
              tunnel: w1126 -> [w1163]
              tunnel: w1125 -> [w1162]
              tunnel: w1124 -> [w1159]
              tunnel: [w1159] -> w1123
              tunnel: w1123 -> [w1238]
              frame #0 {
                n460 = call <vilib>:"Set Busy.vi"() -> ()  [unwired: 10 in, 2 out]
                n461 = property on="Property Node" class="Str"(reference=w1157, "Value"="Updating Motor Parameters\nThis Should Take About 5 Seconds" ("Status Theta")) -> (reference out=w1156:refnum<vi>)  [unwired: 1 in, 1 out]
              }
              frame #1 {
                n462 = call "Motors Status Verbose.vi"("Axis"=1, "VISA in"=w1192, "error in"=w1191) -> ("Slew Speed (mm or deg/s)"=w1208:dbl, "Jogger Normal Speed (mm or deg/s)"=w1209:dbl, "Jogger Fast Speed (mm or deg/s)"=w1210:dbl, "Actual Position (mm or deg)"=w1225:dbl, "OS"=w1199:i32, "Mode"=→"X Action":string, "VISA out"=w1214:refnum<visa-resource-name>, "Creep Speed (mm or deg/s)"=w1181:dbl, "error out"=w1196:errorcluster)  [unwired: 4 in]
                n463 = property on="Property Node" class="DigNum (strict)"(reference=w1182, "Value"=w1208) -> ()  [unwired: 1 in, 2 out]
                n464 = property on="Property Node" class="DigNum (strict)"(reference=w1187, "Value"=w1209) -> ()  [unwired: 1 in, 2 out]
                n465 = property on="Property Node" class="DigNum (strict)"(reference=w1186, "Value"=w1210) -> ()  [unwired: 1 in, 2 out]
                n466 = property on="Property Node" class="DigNum (strict)"(reference=w1185, "Value"=w1225) -> ()  [unwired: 1 in, 2 out]
                n467 = property on="Property Node" class="DigNum (strict)"(reference=w1182, "Minimum"=w1181) -> ()  [unwired: 1 in, 2 out]
                n468 = call "Motors Decipher Status.vi"("OS"=w1199) -> ("Status"=w1235:string)
                n469 = call "Motors Status Verbose.vi"("Axis"=2, "VISA in"=w1214, "error in"=w1196) -> ("Slew Speed (mm or deg/s)"=w1211:dbl, "Jogger Normal Speed (mm or deg/s)"=w1212:dbl, "Jogger Fast Speed (mm or deg/s)"=w1213:dbl, "Actual Position (mm or deg)"=w1226:dbl, "OS"=w1200:i32, "Mode"=→"Y Action":string, "VISA out"=w1215:refnum<visa-resource-name>, "Creep Speed (mm or deg/s)"=w1170:dbl, "error out"=w1197:errorcluster)  [unwired: 4 in]
                n470 = property on="Property Node" class="Str"(reference=w1184, "Value"=w1235) -> ()  [unwired: 1 in, 2 out]
                n471 = property on="Property Node" class="DigNum (strict)"(reference=w1169, "Value"=w1211) -> ()  [unwired: 1 in, 2 out]
                n472 = property on="Property Node" class="DigNum (strict)"(reference=w1180, "Value"=w1212) -> ()  [unwired: 1 in, 2 out]
                n473 = property on="Property Node" class="DigNum (strict)"(reference=w1179, "Value"=w1213) -> ()  [unwired: 1 in, 2 out]
                n474 = property on="Property Node" class="DigNum (strict)"(reference=w1178, "Value"=w1226) -> ()  [unwired: 1 in, 2 out]
                n475 = property on="Property Node" class="DigNum (strict)"(reference=w1169, "Minimum"=w1170) -> ()  [unwired: 1 in, 2 out]
                n476 = call "Motors Status Verbose.vi"("Axis"=3, "VISA in"=w1215, "error in"=w1197) -> ("Slew Speed (mm or deg/s)"=w1224:dbl, "Jogger Normal Speed (mm or deg/s)"=w1223:dbl, "Jogger Fast Speed (mm or deg/s)"=w1222:dbl, "Actual Position (mm or deg)"=w1221:dbl, "OS"=w1201:i32, "Mode"=→"Z Action":string, "VISA out"=w1216:refnum<visa-resource-name>, "Creep Speed (mm or deg/s)"=w1168:dbl, "error out"=w1198:errorcluster)  [unwired: 4 in]
                n477 = call "Motors Decipher Status.vi"("OS"=w1200) -> ("Status"=w1227:string)
                n478 = Not Equal?(x=w1235, y="Idle") -> (x != y?=w1217:bool)
                n479 = property on="Property Node" class="Bool (strict)"(reference=w1183, "Value"=w1217) -> ()  [unwired: 1 in, 2 out]
                n480 = property on="Property Node" class="Str"(reference=w1177, "Value"=w1227) -> ()  [unwired: 1 in, 2 out]
                n481 = property on="Property Node" class="DigNum (strict)"(reference=w1167, "Value"=w1224) -> ()  [unwired: 1 in, 2 out]
                n482 = property on="Property Node" class="DigNum (strict)"(reference=w1175, "Value"=w1223) -> ()  [unwired: 1 in, 2 out]
                n483 = property on="Property Node" class="DigNum (strict)"(reference=w1174, "Value"=w1222) -> ()  [unwired: 1 in, 2 out]
                n484 = property on="Property Node" class="DigNum (strict)"(reference=w1173, "Value"=w1221) -> ()  [unwired: 1 in, 2 out]
                n485 = property on="Property Node" class="DigNum (strict)"(reference=w1167, "Minimum"=w1168) -> ()  [unwired: 1 in, 2 out]
                n486 = call "Motors Status Verbose.vi"("Axis"=4, "VISA in"=w1216, "error in"=w1198) -> ("Slew Speed (mm or deg/s)"=w1230:dbl, "Jogger Normal Speed (mm or deg/s)"=w1231:dbl, "Jogger Fast Speed (mm or deg/s)"=w1232:dbl, "Actual Position (mm or deg)"=w1233:dbl, "OS"=w1202:i32, "Mode"=→"Theta Action":string, "VISA out"=w1190:refnum<visa-resource-name>, "Creep Speed (mm or deg/s)"=w1161:dbl, "error out"=w1189:errorcluster)  [unwired: 4 in]
                n487 = call "Motors Decipher Status.vi"("OS"=w1201) -> ("Status"=w1229:string)
                n488 = Not Equal?(x=w1227, y="Idle") -> (x != y?=w1218:bool)
                n489 = property on="Property Node" class="Bool (strict)"(reference=w1176, "Value"=w1218) -> ()  [unwired: 1 in, 2 out]
                n490 = property on="Property Node" class="Str"(reference=w1172, "Value"=w1229) -> ()  [unwired: 1 in, 2 out]
                n491 = property on="Property Node" class="DigNum (strict)"(reference=w1160, "Value"=w1230) -> ()  [unwired: 1 in, 2 out]
                n492 = property on="Property Node" class="DigNum (strict)"(reference=w1166, "Value"=w1231) -> ()  [unwired: 1 in, 2 out]
                n493 = property on="Property Node" class="DigNum (strict)"(reference=w1165, "Value"=w1232) -> ()  [unwired: 1 in, 2 out]
                n494 = property on="Property Node" class="DigNum (strict)"(reference=w1164, "Value"=w1233) -> ()  [unwired: 1 in, 2 out]
                n495 = property on="Property Node" class="DigNum (strict)"(reference=w1160, "Minimum"=w1161) -> ()  [unwired: 1 in, 2 out]
                n496 = call "Motors Decipher Status.vi"("OS"=w1202) -> ("Status"=w1237:string)
                n497 = Not Equal?(x=w1229, y="Idle") -> (x != y?=w1219:bool)
                n498 = property on="Property Node" class="Bool (strict)"(reference=w1171, "Value"=w1219) -> ()  [unwired: 1 in, 2 out]
                n499 = property on="Property Node" class="Str"(reference=w1163, "Value"=w1237) -> ()  [unwired: 1 in, 2 out]
                n500 = Not Equal?(x=w1237, y="Idle") -> (x != y?=w1220:bool)
                n501 = property on="Property Node" class="Bool (strict)"(reference=w1162, "Value"=w1220) -> ()  [unwired: 1 in, 2 out]
              }
              frame #2 {
                n502 = call <vilib>:"Unset Busy.vi"() -> ()  [unwired: 11 in, 1 out]
                n503 = property on="Property Node" class="Str"(reference=w1238, "Value"="Running" ("Status Theta")) -> ()  [unwired: 1 in, 2 out]
              }
            }
            n504 = property on="Property Node" class="Bool (strict)"(reference=w1149, "Value"=FALSE ("Need to Update Motor Parameters")) -> ()  [unwired: 1 in, 2 out]
          }
        }
        n505 = property on="Property Node" class="Clust (strict)"(reference=w166, "Value"=w447) -> ()  [unwired: 1 in, 2 out]
        "Loop i" <- w440
      }
    }
  }
  n506 = property on="Property Node" class="Clust (strict)"(reference=w2) -> (reference out=w1:refnum<vi>, "Value"=w4:errorcluster)  [unwired: 1 in, 1 out]
  n507 = call "Motors Close.vi"("error in"=w4, "VISA in"=w5) -> ("error out"=w3:errorcluster)  [unwired: 1 in]
  n508 = property on="Property Node" class="Clust (strict)"(reference=w1, "Value"=w3) -> ()  [unwired: 1 in, 2 out]
